vi "4461 - Create IO Channels Parallel Uneven.vi"(1 "Channels: Lockin":T1={"REF f (Hz)"=[0.4, 0.4], "REF phi (°)"=[0.0, 0.0]} {"REF phi (°)" format="%#_3g"}, 4 "sample mode":i32(ring)=10178 items=["Finite Samples"=10178, "Continuous Samples"=10123], 6 "sampling info":cluster{"Fs":dbl, "#s":dbl}, 7 "AI Buffer Size (S)":i32=10, 8 "error in":errorcluster, 9 "AO":T4={"AO amp (V)"=[0.1, 0.09, 0.08, 0.07, 0.06, 0.05, 0.04, 0.03], "AO DC (V)"=[0.0, 0.0, 0.0, 0.0, 0.0, 0.0, 0.0, 0.0], "AO f (Hz)"=[13.0, 13.0, 13.0, 13.0, 13.0, 13.0, 13.0, 13.0], "AO phi (°)"=[0.0, 0.0, 0.0, 0.0, 0.0, 0.0, 0.0, 0.0], "function"=[enum."Sine", enum."Sine", enum."Sine", enum."Sine", enum."Sine", enum."Sine", enum."Sine", enum."Sine"], "I+"=[]} {"AO f (Hz)" min=0.001 max=10000.0; "AO DC (V)" format="%.3p"; "AO amp (V)" format="%.3p"}, 10 "AO Configuration":T11, 11 "AI Configuration":T14) -> (0 "error out":errorcluster, 2 "AO Task":refnum<k21>[](array[refnum]), 3 "AI task":refnum<k21>[](array[refnum]), 5 "phase log":dbl[](array[numeric])=[0.99999999999938, 0.99999999999938])   [LabVIEW 2016]
uses:
  Instrument.Lockin/Typedefs/AI.config-array.ctl
  Instrument.Lockin/Typedefs/AI.config-cluster.ctl
  Instrument.Lockin/Typedefs/AI.coupling-enum.ctl
  Instrument.Lockin/Typedefs/446xAI-enum.ctl
  Instrument.Lockin/Typedefs/AO.config-array.ctl
  Instrument.Lockin/Typedefs/AO.config-cluster.ctl
  Instrument.Lockin/Typedefs/446xAO-enum.ctl
  Instrument.Lockin/Typedefs/AO-cluster.ctl
  Instrument.Lockin/Typedefs/AO_Amp-array.ctl
  Instrument.Lockin/Typedefs/AO_DC-array.ctl
  Instrument.Lockin/Typedefs/AO_f-array.ctl
  Instrument.Lockin/Typedefs/AO_phi-array.ctl
  Instrument.Lockin/Typedefs/Function-array.ctl
  Instrument.Lockin/Typedefs/Function-enum.ctl
  Instrument.Lockin/Typedefs/REF-cluster.ctl
  Instrument.Lockin/Typedefs/REF_f-array.ctl
  Instrument.Lockin/Typedefs/REF_phi-array.ctl
  <vilib>/DAQmx/write.llb/DAQmx Write (Analog 1D Wfm NChan NSamp).vi
  <vilib>/DAQmx/read.llb/DAQmx Read (Analog 1D Wfm NChan NSamp).vi
  <vilib>/DAQmx/create/channels.llb/DAQmx Create Channel (AI-Voltage-Basic).vi
  <vilib>/DAQmx/configure/timing.llb/DAQmx Timing (Sample Clock).vi
  <vilib>/DAQmx/create/channels.llb/DAQmx Create Channel (AO-Voltage-Basic).vi
  <vilib>/DAQmx/configure/trigger.llb/DAQmx Start Trigger (Digital Edge).vi
  <vilib>/DAQmx/miscellaneous.llb/DAQmx Fill In Error Info.vi
  <resource>/objmgr/daqmx.rc
  Instrument.Lockin/Instrument.Lockin.lvclass
panel:
  in  "AI.FilterDelay":dbl
  in  "AI.Gain":dbl
  in  "input terminal configuration":i32(ring)=-1 items=["default"=-1, "RSE"=10083, "NRSE"=10078, "Differential"=10106, "Pseudodifferential"=12529]
  in  "output terminal configuration":i32(ring)=-1 items=["Default"=-1, "RSE"=10083, "Differential"=10106, "Pseudodifferential"=12529]
  in  "SampClk.Timebase.Rate":dbl
  in  "SampQuant.SampPerChan":dbl
  # "1"
  # "2"
  # "3"
  # "4"
  # "5"
  # "6"
  # "7"
  # "8"
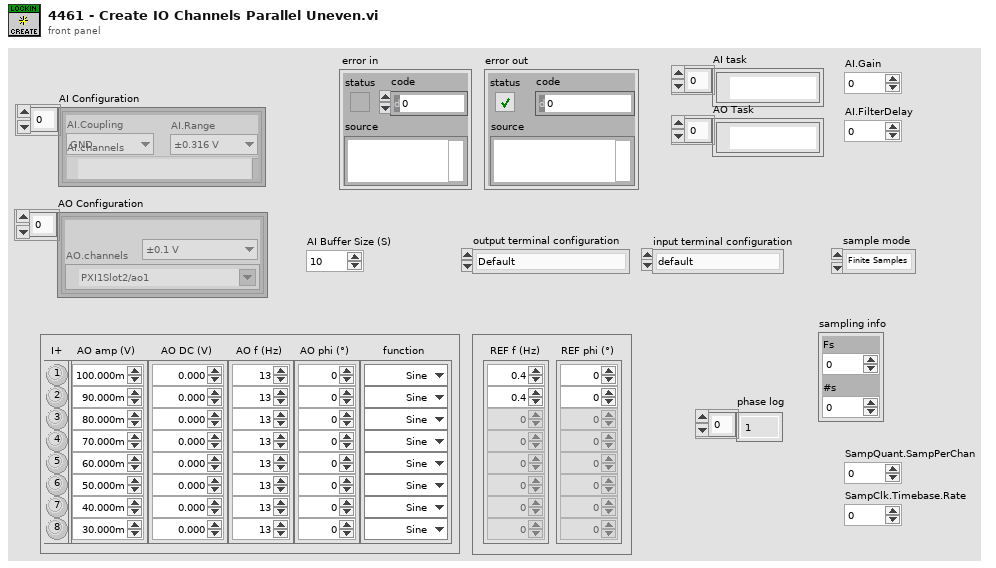
[diagram p1: front panel]
types:
  T1 = typedef "Instrument.Lockin.lvclass/REF-cluster.ctl" = cluster{"REF f (Hz)":T2, "REF phi (°)":T3}
  T2 = typedef "Instrument.Lockin.lvclass/REF_f-array.ctl" = dbl[]
  T3 = typedef "Instrument.Lockin.lvclass/REF_phi-array.ctl" = dbl[]
  T4 = typedef "Instrument.Lockin.lvclass/AO-cluster.ctl" = cluster{"AO amp (V)":T5, "AO DC (V)":T6, "AO f (Hz)":T7, "AO phi (°)":T8, "function":T9, "I+":bool[]}
  T5 = typedef "Instrument.Lockin.lvclass/AO_Amp-array.ctl" = dbl[]
  T6 = typedef "Instrument.Lockin.lvclass/AO_DC-array.ctl" = dbl[]
  T7 = typedef "Instrument.Lockin.lvclass/AO_f-array.ctl" = dbl[]
  T8 = typedef "Instrument.Lockin.lvclass/AO_phi-array.ctl" = dbl[]
  T9 = typedef "Instrument.Lockin.lvclass/Function-array.ctl" = T10[]
  T10 = typedef "Instrument.Lockin.lvclass/Function-enum.ctl" = enum16{"Sine", "Triangle", "Square", "Sawtooth"}
  T11 = typedef "Instrument.Lockin.lvclass/AO.config-array.ctl" = T12[]
  T12 = typedef "Instrument.Lockin.lvclass/AO.config-cluster.ctl" = cluster{"AO.Range":T13, "AO.channels":tag}
  T13 = typedef "Instrument.Lockin.lvclass/446xAO-enum.ctl" = enum16{"±0.1 V", "±1.0 V", "±10.0 V"}
  T14 = typedef "Instrument.Lockin.lvclass/AI.config-array.ctl" = T15[]
  T15 = typedef "Instrument.Lockin.lvclass/AI.config-cluster.ctl" = cluster{"AI.Coupling":T16, "AI.channels":tag, "AI.Range":T17}
  T16 = typedef "Instrument.Lockin.lvclass/AI.coupling-enum.ctl" = enum16{"AC", "DC", "GND"}
  T17 = typedef "Instrument.Lockin.lvclass/446xAI-enum.ctl" = enum16{"±0.316 V", "±1.00 V", "±3.16 V", "±10.0 V", "±31.6 V", "±42.4 V"}
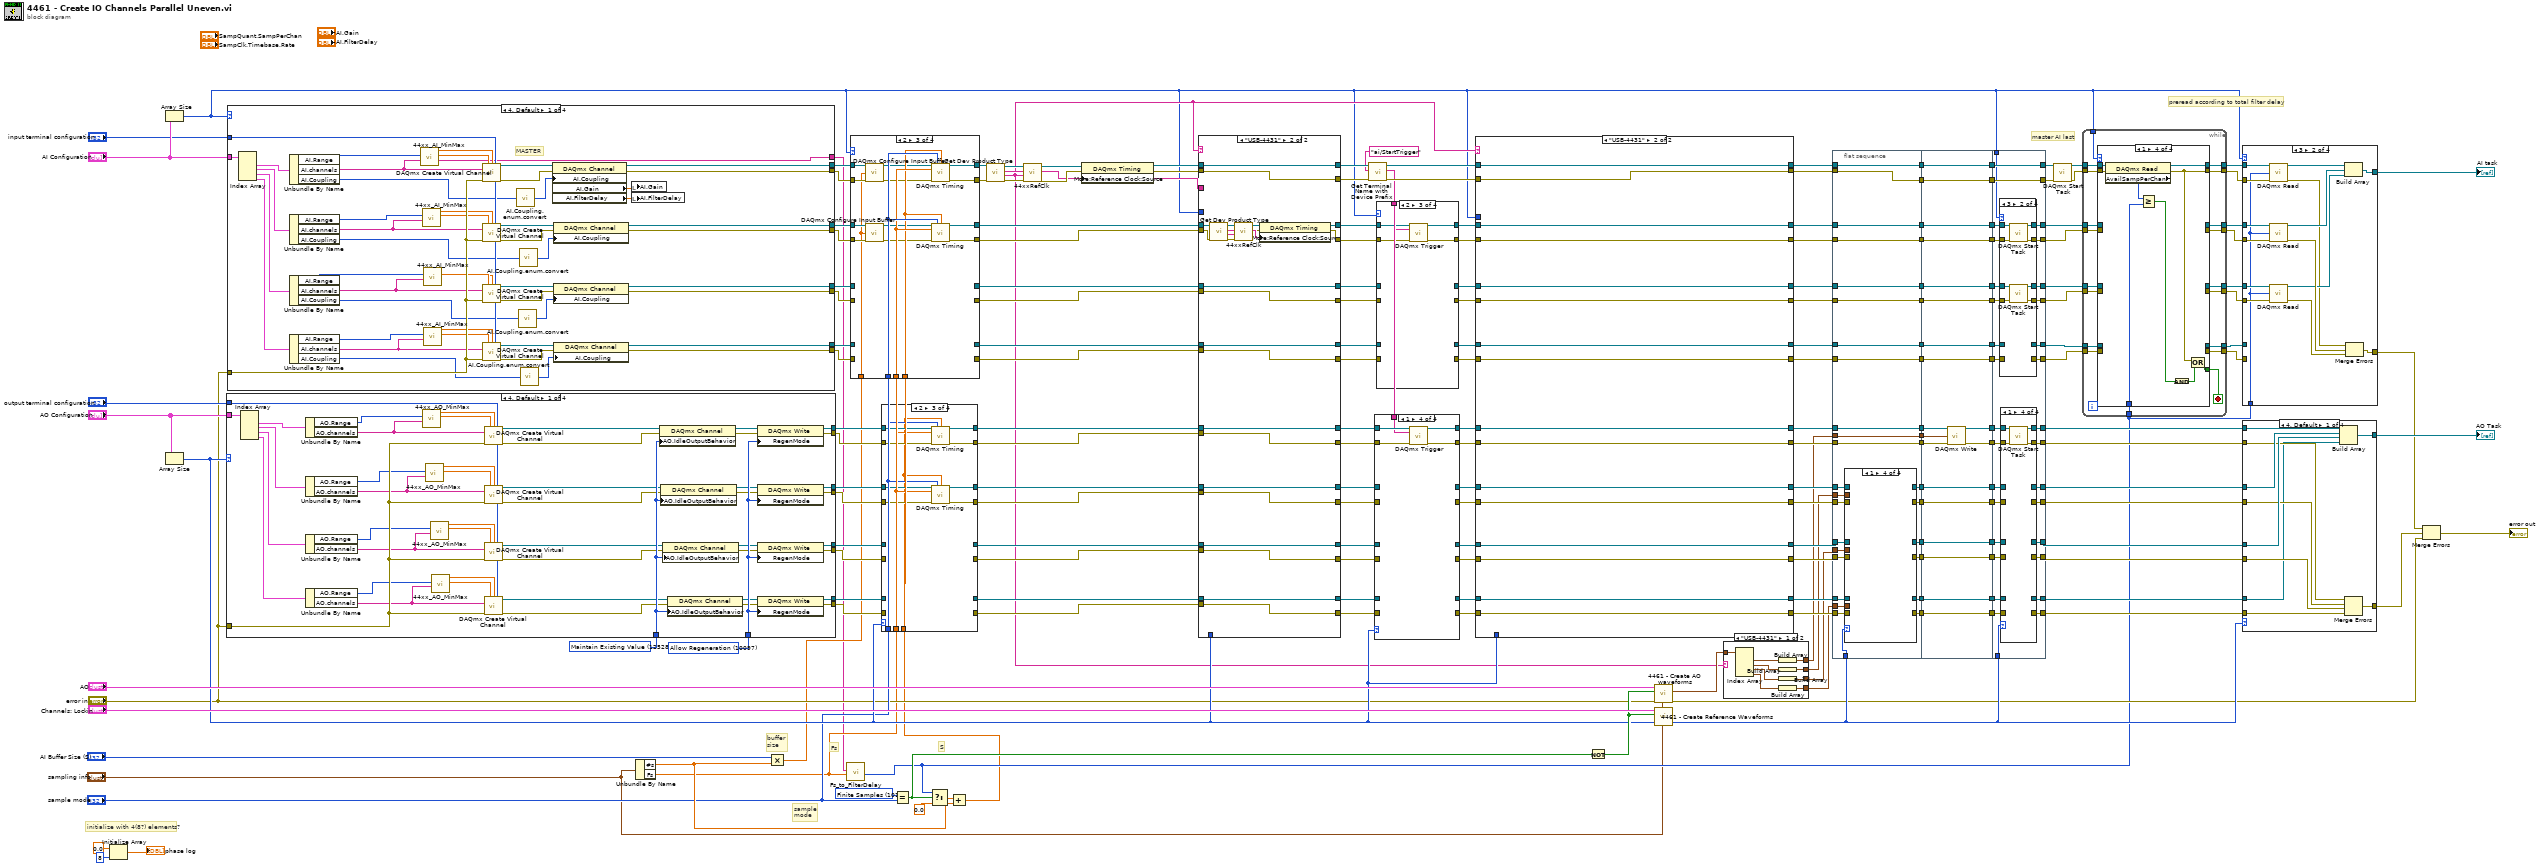
[diagram p0: block diagram]
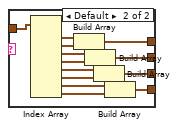
[diagram p2: hidden frame]
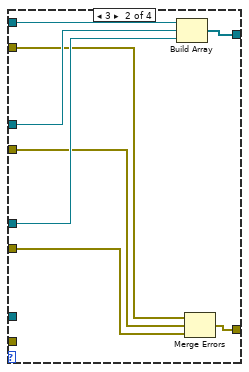
[diagram p3: hidden frame]
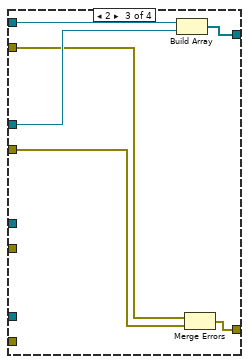
[diagram p4: hidden frame]
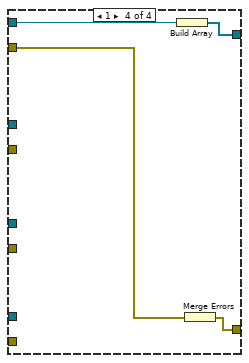
[diagram p5: hidden frame]
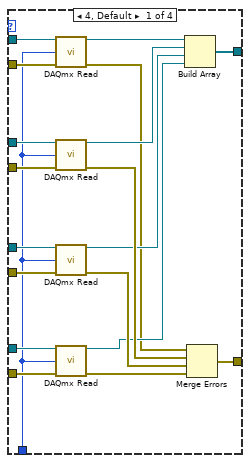
[diagram p6: hidden frame]
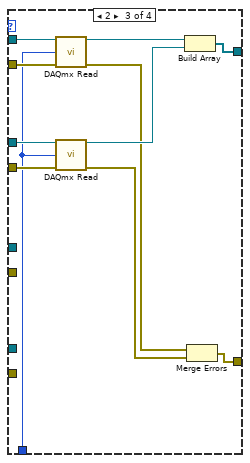
[diagram p7: hidden frame]
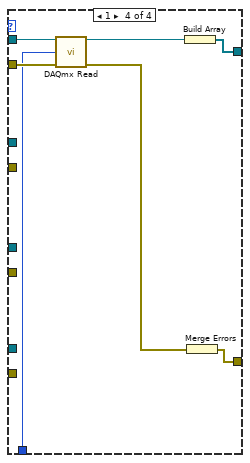
[diagram p8: hidden frame]
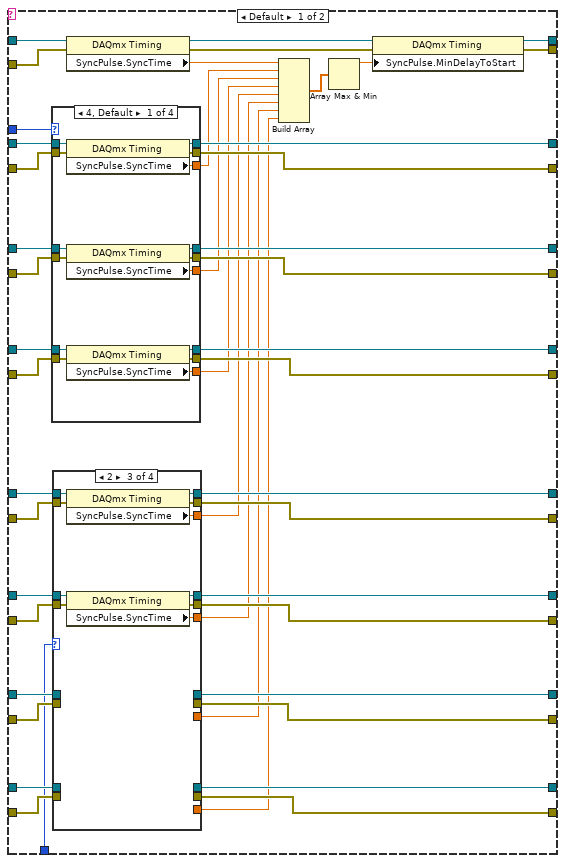
[diagram p9: hidden frame]
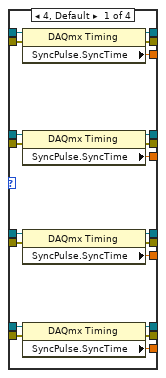
[diagram p10: hidden frame]
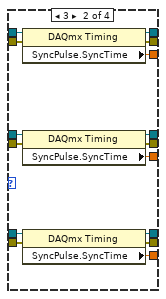
[diagram p11: hidden frame]
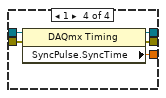
[diagram p12: hidden frame]
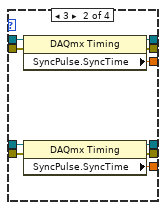
[diagram p13: hidden frame]
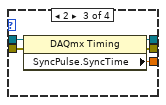
[diagram p14: hidden frame]
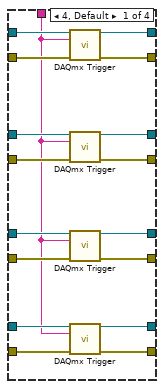
[diagram p16: hidden frame]
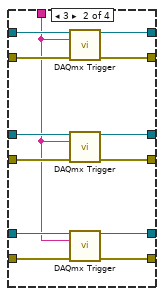
[diagram p17: hidden frame]
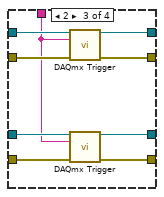
[diagram p18: hidden frame]
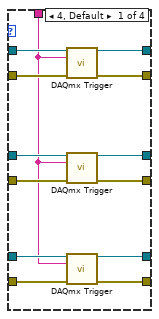
[diagram p19: hidden frame]
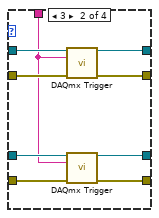
[diagram p20: hidden frame]
diagram:
  w173 = 10097 items=["Allow Regeneration"=10097, "Do Not Allow Regeneration"=10158] ("RegenMode")
  w175 = 12528 items=["Zero Volts"=12526, "High-Impedance"=12527, "Maintain Existing Value"=12528] ("AO.IdleOutputBehavior")
  w177 = 10178 items=["Finite Samples"=10178, "Continuous Samples"=10123] ("sample mode 2")
  # "preread according to total filter delay"
  # "master AI last"
  # "S"
  # "Fs"
  # "sample\nmode"
  # "buffer\nsize"
  # "initialize with 4(8?) elements?"
  n1 = Initialize Array(0.0 ("element"), 8 ("dimension size")) -> (→"phase log":dbl[])
  n2 = Array Size(array="AI Configuration") -> (size(s)=w6:i32)
  n3 = Array Size(array="AO Configuration") -> (size(s)=w168:i32)
  n4 = case shown="4, Default" w168 {
    tunnel: "AO Configuration" -> [w238 w276 w303 w319]
    tunnel: "error in" -> [w206 w251 w285 w308]
    tunnel: "output terminal configuration" -> [w233 w272 w300 w317]
    tunnel: [w228 w267 w295 w312] -> w84
    tunnel: [w227 _ _ _] -> w83
    tunnel: [w226 w266 w294 _] -> w82
    tunnel: [w225 w265 _ _] -> w81
    tunnel: w175 -> [w224 w264 w293 w311]
    tunnel: [w223 w263 w292 w310] -> w72
    tunnel: [w222 w262 w291 _] -> w71
    tunnel: [w221 w261 _ _] -> w70
    tunnel: [w220 _ _ _] -> w69
    tunnel: w173 -> [w219 w260 w290 w309]
    frame 4, Default {
      n5 = Index Array(array=w238) -> (element #1=w237:T12, element #2=w234:T12, element #3=w235:T12, element #4=w236:T12)  [unwired: 4 in]
      n6 = Unbundle By Name(w237) -> ("AO.Range"=w205:T13, "AO.channels"=w193:tag)
      n7 = Unbundle By Name(w234) -> ("AO.Range"=w200:T13, "AO.channels"=w192:tag)
      n8 = Unbundle By Name(w235) -> ("AO.Range"=w201:T13, "AO.channels"=w191:tag)
      n9 = Unbundle By Name(w236) -> ("AO.Range"=w202:T13, "AO.channels"=w190:tag)
      n10 = call "44xx_AO_MinMax.vi"("AO.channels"=w193, "AO.Range"=w205) -> ("AO.max"=w204:dbl, "AO.min"=w203:dbl)  [unwired: 7 in, 1 out]
      n11 = call "44xx_AO_MinMax.vi"("AO.channels"=w192, "AO.Range"=w200) -> ("AO.max"=w199:dbl, "AO.min"=w198:dbl)  [unwired: 7 in, 1 out]
      n12 = call "44xx_AO_MinMax.vi"("AO.channels"=w191, "AO.Range"=w201) -> ("AO.max"=w197:dbl, "AO.min"=w196:dbl)  [unwired: 7 in, 1 out]
      n13 = call "44xx_AO_MinMax.vi"("AO.channels"=w190, "AO.Range"=w202) -> ("AO.max"=w195:dbl, "AO.min"=w194:dbl)  [unwired: 7 in, 1 out]
      n14 = call-poly <vilib>:"DAQmx Create Virtual Channel.vi"("maximum value"=w204, "minimum value"=w203, "output terminal configuration"=w233, "physical channels"=w193, "error in"=w206) -> ("task out"=w232:refnum<k21>, "error out"=w231:errorcluster)  [unwired: 9 in]
      n15 = call-poly <vilib>:"DAQmx Create Virtual Channel.vi"("maximum value"=w199, "minimum value"=w198, "output terminal configuration"=w233, "physical channels"=w192, "error in"=w206) -> ("task out"=w213:refnum<k21>, "error out"=w214:errorcluster)  [unwired: 9 in]
      n16 = call-poly <vilib>:"DAQmx Create Virtual Channel.vi"("maximum value"=w197, "minimum value"=w196, "output terminal configuration"=w233, "physical channels"=w191, "error in"=w206) -> ("task out"=w215:refnum<k21>, "error out"=w216:errorcluster)  [unwired: 9 in]
      n17 = call-poly <vilib>:"DAQmx Create Virtual Channel.vi"("maximum value"=w195, "minimum value"=w194, "output terminal configuration"=w233, "physical channels"=w190, "error in"=w206) -> ("task out"=w218:refnum<k21>, "error out"=w217:errorcluster)  [unwired: 9 in]
      n18 = property class="DAQmx Channel"(reference=w232, error in=w231, "AO.IdleOutputBehavior"=w224) -> (reference out=w230:refnum<k21>, error out=w229:errorcluster)
      n19 = property class="DAQmx Channel"(reference=w213, error in=w214, "AO.IdleOutputBehavior"=w224) -> (reference out=w207:refnum<k21>, error out=w208:errorcluster)
      n20 = property class="DAQmx Channel"(reference=w215, error in=w216, "AO.IdleOutputBehavior"=w224) -> (reference out=w209:refnum<k21>, error out=w210:errorcluster)
      n21 = property class="DAQmx Channel"(reference=w218, error in=w217, "AO.IdleOutputBehavior"=w224) -> (reference out=w212:refnum<k21>, error out=w211:errorcluster)
      n22 = property class="DAQmx Write"(reference=w230, error in=w229, "RegenMode"=w219) -> (reference out=w228:refnum<k21>, error out=w223:errorcluster)
      n23 = property class="DAQmx Write"(reference=w207, error in=w208, "RegenMode"=w219) -> (reference out=w226:refnum<k21>, error out=w222:errorcluster)
      n24 = property class="DAQmx Write"(reference=w209, error in=w210, "RegenMode"=w219) -> (reference out=w225:refnum<k21>, error out=w221:errorcluster)
      n25 = property class="DAQmx Write"(reference=w212, error in=w211, "RegenMode"=w219) -> (reference out=w227:refnum<k21>, error out=w220:errorcluster)
    }
    frame 3 {
      n26 = Index Array(array=w276) -> (element #1=w275:T12, element #2=w273:T12, element #3=w274:T12)  [unwired: 4 in, 1 out]
      n27 = Unbundle By Name(w275) -> ("AO.Range"=w250:T13, "AO.channels"=w239:tag)
      n28 = Unbundle By Name(w273) -> ("AO.Range"=w246:T13, "AO.channels"=w240:tag)
      n29 = Unbundle By Name(w274) -> ("AO.Range"=w247:T13, "AO.channels"=w241:tag)
      n30 = call "44xx_AO_MinMax.vi"("AO.channels"=w239, "AO.Range"=w250) -> ("AO.max"=w249:dbl, "AO.min"=w248:dbl)  [unwired: 7 in, 1 out]
      n31 = call "44xx_AO_MinMax.vi"("AO.channels"=w240, "AO.Range"=w246) -> ("AO.max"=w245:dbl, "AO.min"=w244:dbl)  [unwired: 7 in, 1 out]
      n32 = call "44xx_AO_MinMax.vi"("AO.channels"=w241, "AO.Range"=w247) -> ("AO.max"=w243:dbl, "AO.min"=w242:dbl)  [unwired: 7 in, 1 out]
      n33 = call-poly <vilib>:"DAQmx Create Virtual Channel.vi"("maximum value"=w249, "minimum value"=w248, "output terminal configuration"=w272, "physical channels"=w239, "error in"=w251) -> ("task out"=w271:refnum<k21>, "error out"=w270:errorcluster)  [unwired: 9 in]
      n34 = call-poly <vilib>:"DAQmx Create Virtual Channel.vi"("maximum value"=w245, "minimum value"=w244, "output terminal configuration"=w272, "physical channels"=w240, "error in"=w251) -> ("task out"=w256:refnum<k21>, "error out"=w257:errorcluster)  [unwired: 9 in]
      n35 = call-poly <vilib>:"DAQmx Create Virtual Channel.vi"("maximum value"=w243, "minimum value"=w242, "output terminal configuration"=w272, "physical channels"=w241, "error in"=w251) -> ("task out"=w258:refnum<k21>, "error out"=w259:errorcluster)  [unwired: 9 in]
      n36 = property class="DAQmx Channel"(reference=w271, error in=w270, "AO.IdleOutputBehavior"=w264) -> (reference out=w269:refnum<k21>, error out=w268:errorcluster)
      n37 = property class="DAQmx Channel"(reference=w256, error in=w257, "AO.IdleOutputBehavior"=w264) -> (reference out=w252:refnum<k21>, error out=w253:errorcluster)
      n38 = property class="DAQmx Channel"(reference=w258, error in=w259, "AO.IdleOutputBehavior"=w264) -> (reference out=w254:refnum<k21>, error out=w255:errorcluster)
      n39 = property class="DAQmx Write"(reference=w269, error in=w268, "RegenMode"=w260) -> (reference out=w267:refnum<k21>, error out=w263:errorcluster)
      n40 = property class="DAQmx Write"(reference=w252, error in=w253, "RegenMode"=w260) -> (reference out=w266:refnum<k21>, error out=w262:errorcluster)
      n41 = property class="DAQmx Write"(reference=w254, error in=w255, "RegenMode"=w260) -> (reference out=w265:refnum<k21>, error out=w261:errorcluster)
    }
    frame 2 {
      n42 = Index Array(array=w303) -> (element #1=w302:T12, element #2=w301:T12)  [unwired: 4 in, 2 out]
      n43 = Unbundle By Name(w302) -> ("AO.Range"=w284:T13, "AO.channels"=w278:tag)
      n44 = Unbundle By Name(w301) -> ("AO.Range"=w281:T13, "AO.channels"=w277:tag)
      n45 = call "44xx_AO_MinMax.vi"("AO.channels"=w278, "AO.Range"=w284) -> ("AO.max"=w283:dbl, "AO.min"=w282:dbl)  [unwired: 7 in, 1 out]
      n46 = call "44xx_AO_MinMax.vi"("AO.channels"=w277, "AO.Range"=w281) -> ("AO.max"=w280:dbl, "AO.min"=w279:dbl)  [unwired: 7 in, 1 out]
      n47 = call-poly <vilib>:"DAQmx Create Virtual Channel.vi"("maximum value"=w283, "minimum value"=w282, "output terminal configuration"=w300, "physical channels"=w278, "error in"=w285) -> ("task out"=w299:refnum<k21>, "error out"=w298:errorcluster)  [unwired: 9 in]
      n48 = call-poly <vilib>:"DAQmx Create Virtual Channel.vi"("maximum value"=w280, "minimum value"=w279, "output terminal configuration"=w300, "physical channels"=w277, "error in"=w285) -> ("task out"=w288:refnum<k21>, "error out"=w289:errorcluster)  [unwired: 9 in]
      n49 = property class="DAQmx Channel"(reference=w299, error in=w298, "AO.IdleOutputBehavior"=w293) -> (reference out=w297:refnum<k21>, error out=w296:errorcluster)
      n50 = property class="DAQmx Channel"(reference=w288, error in=w289, "AO.IdleOutputBehavior"=w293) -> (reference out=w286:refnum<k21>, error out=w287:errorcluster)
      n51 = property class="DAQmx Write"(reference=w297, error in=w296, "RegenMode"=w290) -> (reference out=w295:refnum<k21>, error out=w292:errorcluster)
      n52 = property class="DAQmx Write"(reference=w286, error in=w287, "RegenMode"=w290) -> (reference out=w294:refnum<k21>, error out=w291:errorcluster)
    }
    frame 1 {
      n53 = Index Array(array=w319) -> (element #1=w318:T12)  [unwired: 4 in, 3 out]
      n54 = Unbundle By Name(w318) -> ("AO.Range"=w305:T13, "AO.channels"=w304:tag)
      n55 = call "44xx_AO_MinMax.vi"("AO.channels"=w304, "AO.Range"=w305) -> ("AO.max"=w307:dbl, "AO.min"=w306:dbl)  [unwired: 7 in, 1 out]
      n56 = call-poly <vilib>:"DAQmx Create Virtual Channel.vi"("maximum value"=w307, "minimum value"=w306, "output terminal configuration"=w317, "physical channels"=w304, "error in"=w308) -> ("task out"=w316:refnum<k21>, "error out"=w315:errorcluster)  [unwired: 9 in]
      n57 = property class="DAQmx Channel"(reference=w316, error in=w315, "AO.IdleOutputBehavior"=w311) -> (reference out=w314:refnum<k21>, error out=w313:errorcluster)
      n58 = property class="DAQmx Write"(reference=w314, error in=w313, "RegenMode"=w309) -> (reference out=w312:refnum<k21>, error out=w310:errorcluster)
    }
  }
  n59 = case shown="4, Default" w6 {
    tunnel: "AI Configuration" -> [w369 w408 w436 w453]
    tunnel: "error in" -> [w368 w407 w435 w452]
    tunnel: "input terminal configuration" -> [w367 w406 w434 w451]
    tunnel: [w366 w405 w433 _] -> w75
    tunnel: [w365 w404 _ _] -> w74
    tunnel: [w364 _ _ _] -> w73
    tunnel: [w363 w403 w432 _] -> w18
    tunnel: [w362 w402 _ _] -> w17
    tunnel: [w361 _ _ _] -> w16
    tunnel: [w360 w401 w431 w450] -> w48
    tunnel: [w359 w400 w430 w449] -> w19
    tunnel: [w320 w370 w409 w437] -> w2
    frame 4, Default {
      # "MASTER"
      n60 = Index Array(array=w369) -> (element #1=w334:T15, element #2=w356:T15, element #3=w355:T15, element #4=w354:T15)  [unwired: 4 in]
      n61 = Unbundle By Name(w334) -> ("AI.Range"=w335:T17, "AI.channels"=w326:tag, "AI.Coupling"=w351:T16)
      n62 = Unbundle By Name(w356) -> ("AI.Range"=w324:T17, "AI.channels"=w325:tag, "AI.Coupling"=w342:T16)
      n63 = Unbundle By Name(w355) -> ("AI.Range"=w333:T17, "AI.channels"=w323:tag, "AI.Coupling"=w343:T16)
      n64 = Unbundle By Name(w354) -> ("AI.Range"=w322:T17, "AI.channels"=w321:tag, "AI.Coupling"=w344:T16)
      n65 = call "44xx_AI_MinMax.vi"("AI.channels"=w326, "446x AI"=w335) -> ("ProductType"=w320:string, "AI.Max"=w337:dbl, "AI.Min"=w336:dbl)  [unwired: 7 in]
      n66 = call "44xx_AI_MinMax.vi"("AI.channels"=w325, "446x AI"=w324) -> ("AI.Max"=w332:dbl, "AI.Min"=w329:dbl)  [unwired: 7 in, 1 out]
      n67 = call "44xx_AI_MinMax.vi"("AI.channels"=w321, "446x AI"=w322) -> ("AI.Max"=w328:dbl, "AI.Min"=w327:dbl)  [unwired: 7 in, 1 out]
      n68 = call "44xx_AI_MinMax.vi"("AI.channels"=w323, "446x AI"=w333) -> ("AI.Max"=w331:dbl, "AI.Min"=w330:dbl)  [unwired: 7 in, 1 out]
      n69 = call-poly <vilib>:"DAQmx Create Virtual Channel.vi"("maximum value"=w337, "minimum value"=w336, "input terminal configuration"=w367, "physical channels"=w326, "error in"=w368) -> ("task out"=w358:refnum<k21>, "error out"=w357:errorcluster)  [unwired: 9 in]
      n70 = call-poly <vilib>:"DAQmx Create Virtual Channel.vi"("maximum value"=w332, "minimum value"=w329, "input terminal configuration"=w367, "physical channels"=w325, "error in"=w368) -> ("task out"=w349:refnum<k21>, "error out"=w350:errorcluster)  [unwired: 9 in]
      n71 = call-poly <vilib>:"DAQmx Create Virtual Channel.vi"("maximum value"=w331, "minimum value"=w330, "input terminal configuration"=w367, "physical channels"=w323, "error in"=w368) -> ("task out"=w348:refnum<k21>, "error out"=w347:errorcluster)  [unwired: 9 in]
      n72 = call-poly <vilib>:"DAQmx Create Virtual Channel.vi"("maximum value"=w328, "minimum value"=w327, "input terminal configuration"=w367, "physical channels"=w321, "error in"=w368) -> ("task out"=w345:refnum<k21>, "error out"=w346:errorcluster)  [unwired: 9 in]
      n73 = call "AI.Coupling.enum.convert.vi"("AI.Coupling"=w351) -> ("Numeric"=w341:i32)
      n74 = call "AI.Coupling.enum.convert.vi"("AI.Coupling"=w343) -> ("Numeric"=w339:i32)
      n75 = call "AI.Coupling.enum.convert.vi"("AI.Coupling"=w342) -> ("Numeric"=w340:i32)
      n76 = call "AI.Coupling.enum.convert.vi"("AI.Coupling"=w344) -> ("Numeric"=w338:i32)
      n77 = property class="DAQmx Channel"(reference=w358, error in=w357, "AI.Coupling"=w341) -> (reference out=w360:refnum<k21>, error out=w359:errorcluster, "AI.Gain"=w353:dbl, "AI.FilterDelay"=w352:dbl)
      n78 = property class="DAQmx Channel"(reference=w349, error in=w350, "AI.Coupling"=w340) -> (reference out=w366:refnum<k21>, error out=w363:errorcluster)
      n79 = property class="DAQmx Channel"(reference=w348, error in=w347, "AI.Coupling"=w339) -> (reference out=w365:refnum<k21>, error out=w362:errorcluster)
      n80 = property class="DAQmx Channel"(reference=w345, error in=w346, "AI.Coupling"=w338) -> (reference out=w364:refnum<k21>, error out=w361:errorcluster)
      n81 = local write "AI.Gain"(w353) -> ()
      n82 = local write "AI.FilterDelay"(w352) -> ()
    }
    frame 3 {
      # "MASTER"
      n83 = Index Array(array=w408) -> (element #1=w380:T15, element #2=w397:T15, element #3=w396:T15)  [unwired: 4 in, 1 out]
      n84 = Unbundle By Name(w380) -> ("AI.Range"=w381:T17, "AI.channels"=w371:tag, "AI.Coupling"=w393:T16)
      n85 = Unbundle By Name(w397) -> ("AI.Range"=w372:T17, "AI.channels"=w373:tag, "AI.Coupling"=w387:T16)
      n86 = Unbundle By Name(w396) -> ("AI.Range"=w379:T17, "AI.channels"=w374:tag, "AI.Coupling"=w388:T16)
      n87 = call "44xx_AI_MinMax.vi"("AI.channels"=w371, "446x AI"=w381) -> ("ProductType"=w370:string, "AI.Max"=w383:dbl, "AI.Min"=w382:dbl)  [unwired: 7 in]
      n88 = call "44xx_AI_MinMax.vi"("AI.channels"=w373, "446x AI"=w372) -> ("AI.Max"=w378:dbl, "AI.Min"=w375:dbl)  [unwired: 7 in, 1 out]
      n89 = call "44xx_AI_MinMax.vi"("AI.channels"=w374, "446x AI"=w379) -> ("AI.Max"=w377:dbl, "AI.Min"=w376:dbl)  [unwired: 7 in, 1 out]
      n90 = call-poly <vilib>:"DAQmx Create Virtual Channel.vi"("maximum value"=w383, "minimum value"=w382, "input terminal configuration"=w406, "physical channels"=w371, "error in"=w407) -> ("task out"=w399:refnum<k21>, "error out"=w398:errorcluster)  [unwired: 9 in]
      n91 = call-poly <vilib>:"DAQmx Create Virtual Channel.vi"("maximum value"=w378, "minimum value"=w375, "input terminal configuration"=w406, "physical channels"=w373, "error in"=w407) -> ("task out"=w391:refnum<k21>, "error out"=w392:errorcluster)  [unwired: 9 in]
      n92 = call-poly <vilib>:"DAQmx Create Virtual Channel.vi"("maximum value"=w377, "minimum value"=w376, "input terminal configuration"=w406, "physical channels"=w374, "error in"=w407) -> ("task out"=w390:refnum<k21>, "error out"=w389:errorcluster)  [unwired: 9 in]
      n93 = call "AI.Coupling.enum.convert.vi"("AI.Coupling"=w393) -> ("Numeric"=w386:i32)
      n94 = call "AI.Coupling.enum.convert.vi"("AI.Coupling"=w388) -> ("Numeric"=w384:i32)
      n95 = call "AI.Coupling.enum.convert.vi"("AI.Coupling"=w387) -> ("Numeric"=w385:i32)
      n96 = property class="DAQmx Channel"(reference=w399, error in=w398, "AI.Coupling"=w386) -> (reference out=w401:refnum<k21>, error out=w400:errorcluster, "AI.Gain"=w395:dbl, "AI.FilterDelay"=w394:dbl)
      n97 = property class="DAQmx Channel"(reference=w391, error in=w392, "AI.Coupling"=w385) -> (reference out=w405:refnum<k21>, error out=w403:errorcluster)
      n98 = property class="DAQmx Channel"(reference=w390, error in=w389, "AI.Coupling"=w384) -> (reference out=w404:refnum<k21>, error out=w402:errorcluster)
      n99 = local write "AI.Gain"(w395) -> ()
      n100 = local write "AI.FilterDelay"(w394) -> ()
    }
    frame 2 {
      # "MASTER"
      n101 = Index Array(array=w436) -> (element #1=w415:T15, element #2=w427:T15)  [unwired: 4 in, 2 out]
      n102 = Unbundle By Name(w415) -> ("AI.Range"=w416:T17, "AI.channels"=w410:tag, "AI.Coupling"=w424:T16)
      n103 = Unbundle By Name(w427) -> ("AI.Range"=w412:T17, "AI.channels"=w411:tag, "AI.Coupling"=w421:T16)
      n104 = call "44xx_AI_MinMax.vi"("AI.channels"=w410, "446x AI"=w416) -> ("ProductType"=w409:string, "AI.Max"=w418:dbl, "AI.Min"=w417:dbl)  [unwired: 7 in]
      n105 = call "44xx_AI_MinMax.vi"("AI.channels"=w411, "446x AI"=w412) -> ("AI.Max"=w414:dbl, "AI.Min"=w413:dbl)  [unwired: 7 in, 1 out]
      n106 = call-poly <vilib>:"DAQmx Create Virtual Channel.vi"("maximum value"=w418, "minimum value"=w417, "input terminal configuration"=w434, "physical channels"=w410, "error in"=w435) -> ("task out"=w429:refnum<k21>, "error out"=w428:errorcluster)  [unwired: 9 in]
      n107 = call-poly <vilib>:"DAQmx Create Virtual Channel.vi"("maximum value"=w414, "minimum value"=w413, "input terminal configuration"=w434, "physical channels"=w411, "error in"=w435) -> ("task out"=w422:refnum<k21>, "error out"=w423:errorcluster)  [unwired: 9 in]
      n108 = call "AI.Coupling.enum.convert.vi"("AI.Coupling"=w424) -> ("Numeric"=w420:i32)
      n109 = call "AI.Coupling.enum.convert.vi"("AI.Coupling"=w421) -> ("Numeric"=w419:i32)
      n110 = property class="DAQmx Channel"(reference=w429, error in=w428, "AI.Coupling"=w420) -> (reference out=w431:refnum<k21>, error out=w430:errorcluster, "AI.Gain"=w426:dbl, "AI.FilterDelay"=w425:dbl)
      n111 = property class="DAQmx Channel"(reference=w422, error in=w423, "AI.Coupling"=w419) -> (reference out=w433:refnum<k21>, error out=w432:errorcluster)
      n112 = local write "AI.Gain"(w426) -> ()
      n113 = local write "AI.FilterDelay"(w425) -> ()
    }
    frame 1 {
      # "MASTER"
      n114 = Index Array(array=w453) -> (element #1=w442:T15)  [unwired: 4 in, 3 out]
      n115 = Unbundle By Name(w442) -> ("AI.Range"=w441:T17, "AI.channels"=w440:tag, "AI.Coupling"=w444:T16)
      n116 = call "44xx_AI_MinMax.vi"("AI.channels"=w440, "446x AI"=w441) -> ("ProductType"=w437:string, "AI.Max"=w439:dbl, "AI.Min"=w438:dbl)  [unwired: 7 in]
      n117 = call-poly <vilib>:"DAQmx Create Virtual Channel.vi"("maximum value"=w439, "minimum value"=w438, "input terminal configuration"=w451, "physical channels"=w440, "error in"=w452) -> ("task out"=w448:refnum<k21>, "error out"=w447:errorcluster)  [unwired: 9 in]
      n118 = call "AI.Coupling.enum.convert.vi"("AI.Coupling"=w444) -> ("Numeric"=w443:i32)
      n119 = property class="DAQmx Channel"(reference=w448, error in=w447, "AI.Coupling"=w443) -> (reference out=w450:refnum<k21>, error out=w449:errorcluster, "AI.Gain"=w446:dbl, "AI.FilterDelay"=w445:dbl)
      n120 = local write "AI.Gain"(w446) -> ()
      n121 = local write "AI.FilterDelay"(w445) -> ()
    }
  }
  n122 = Unbundle By Name("sampling info") -> ("#s"=w174:dbl, "Fs"=w5:dbl)
  n123 = Multiply(x="AI Buffer Size (S)", y=w174) -> (x*y=w20:dbl)
  n124 = call "Fs_to_FilterDelay.vi"("Fs"=w5, "ProductType"=w2) -> ("Total Filter Delay (samples)"=w4:u32)  [unwired: 9 in]
  n125 = Equal?(x=w177, y="sample mode") -> (x = y?=w171:bool)
  n126 = Select(t=w4, s=w171, f=0.0) -> (s? t:f=w178:dbl)
  n127 = Add(x=w178, y=w174) -> (x+y=w3:dbl)
  n128 = case shown="2" w6 {
    tunnel: [w481 w503 w519 w529] -> w14
    tunnel: [w480 w502 w518 w528] -> w15
    tunnel: [w479 w501 w517 _] -> w131
    tunnel: [w478 w500 w516 _] -> w130
    tunnel: [w477 w499 _ _] -> w125
    tunnel: [w476 w498 _ _] -> w124
    tunnel: [w475 _ _ _] -> w123
    tunnel: [w474 _ _ _] -> w122
    tunnel: w73 -> [w464 _ _ _]
    tunnel: w74 -> [w466 w490 _ _]
    tunnel: w17 -> [w459 w487 _ _]
    tunnel: w16 -> [w465 _ _ _]
    tunnel: w18 -> [w468 w492 w510 _]
    tunnel: w75 -> [w467 w491 w509 _]
    tunnel: "sample mode" -> [w473 w497 w515 w527]
    tunnel: w5 -> [w472 w496 w514 w526]
    tunnel: w3 -> [w471 w495 w513 w525]
    tunnel: w19 -> [w470 w494 w512 w524]
    tunnel: w48 -> [w469 w493 w511 w523]
    tunnel: w20 -> [w454 w482 w504 w520]
    frame 4, Default {
      n129 = call <vilib>:"DAQmx Configure Input Buffer.vi"("task/channels in"=w469, "buffer size (in samples per channel)"=w454, "error in"=w470) -> ("task out"=w455:refnum<k21>, "error out"=w456:errorcluster)  [unwired: 11 in]
      n130 = call <vilib>:"DAQmx Configure Input Buffer.vi"("task/channels in"=w467, "buffer size (in samples per channel)"=w454, "error in"=w468) -> ("task out"=w457:refnum<k21>, "error out"=w458:errorcluster)  [unwired: 11 in]
      n131 = call <vilib>:"DAQmx Configure Input Buffer.vi"("task/channels in"=w466, "buffer size (in samples per channel)"=w454, "error in"=w459) -> ("task out"=w460:refnum<k21>, "error out"=w461:errorcluster)  [unwired: 11 in]
      n132 = call <vilib>:"DAQmx Configure Input Buffer.vi"("task/channels in"=w464, "buffer size (in samples per channel)"=w454, "error in"=w465) -> ("task out"=w463:refnum<k21>, "error out"=w462:errorcluster)  [unwired: 11 in]
      n133 = call-poly <vilib>:"DAQmx Timing.vi"("task/channels in"=w455, "sample mode"=w473, "samples per channel"=w471, "rate"=w472, "error in"=w456) -> ("task out"=w481:refnum<k21>, "error out"=w480:errorcluster)  [unwired: 9 in]
      n134 = call-poly <vilib>:"DAQmx Timing.vi"("task/channels in"=w457, "sample mode"=w473, "samples per channel"=w471, "rate"=w472, "error in"=w458) -> ("task out"=w479:refnum<k21>, "error out"=w478:errorcluster)  [unwired: 9 in]
      n135 = call-poly <vilib>:"DAQmx Timing.vi"("task/channels in"=w460, "sample mode"=w473, "samples per channel"=w471, "rate"=w472, "error in"=w461) -> ("task out"=w476:refnum<k21>, "error out"=w477:errorcluster)  [unwired: 9 in]
      n136 = call-poly <vilib>:"DAQmx Timing.vi"("task/channels in"=w463, "sample mode"=w473, "samples per channel"=w471, "rate"=w472, "error in"=w462) -> ("task out"=w475:refnum<k21>, "error out"=w474:errorcluster)  [unwired: 9 in]
    }
    frame 3 {
      n137 = call <vilib>:"DAQmx Configure Input Buffer.vi"("task/channels in"=w493, "buffer size (in samples per channel)"=w482, "error in"=w494) -> ("task out"=w483:refnum<k21>, "error out"=w484:errorcluster)  [unwired: 11 in]
      n138 = call <vilib>:"DAQmx Configure Input Buffer.vi"("task/channels in"=w491, "buffer size (in samples per channel)"=w482, "error in"=w492) -> ("task out"=w485:refnum<k21>, "error out"=w486:errorcluster)  [unwired: 11 in]
      n139 = call <vilib>:"DAQmx Configure Input Buffer.vi"("task/channels in"=w490, "buffer size (in samples per channel)"=w482, "error in"=w487) -> ("task out"=w488:refnum<k21>, "error out"=w489:errorcluster)  [unwired: 11 in]
      n140 = call-poly <vilib>:"DAQmx Timing.vi"("task/channels in"=w483, "sample mode"=w497, "samples per channel"=w495, "rate"=w496, "error in"=w484) -> ("task out"=w503:refnum<k21>, "error out"=w502:errorcluster)  [unwired: 9 in]
      n141 = call-poly <vilib>:"DAQmx Timing.vi"("task/channels in"=w485, "sample mode"=w497, "samples per channel"=w495, "rate"=w496, "error in"=w486) -> ("task out"=w501:refnum<k21>, "error out"=w500:errorcluster)  [unwired: 9 in]
      n142 = call-poly <vilib>:"DAQmx Timing.vi"("task/channels in"=w488, "sample mode"=w497, "samples per channel"=w495, "rate"=w496, "error in"=w489) -> ("task out"=w498:refnum<k21>, "error out"=w499:errorcluster)  [unwired: 9 in]
    }
    frame 2 {
      n143 = call <vilib>:"DAQmx Configure Input Buffer.vi"("task/channels in"=w511, "buffer size (in samples per channel)"=w504, "error in"=w512) -> ("task out"=w505:refnum<k21>, "error out"=w506:errorcluster)  [unwired: 11 in]
      n144 = call <vilib>:"DAQmx Configure Input Buffer.vi"("task/channels in"=w509, "buffer size (in samples per channel)"=w504, "error in"=w510) -> ("task out"=w507:refnum<k21>, "error out"=w508:errorcluster)  [unwired: 11 in]
      n145 = call-poly <vilib>:"DAQmx Timing.vi"("task/channels in"=w505, "sample mode"=w515, "samples per channel"=w513, "rate"=w514, "error in"=w506) -> ("task out"=w519:refnum<k21>, "error out"=w518:errorcluster)  [unwired: 9 in]
      n146 = call-poly <vilib>:"DAQmx Timing.vi"("task/channels in"=w507, "sample mode"=w515, "samples per channel"=w513, "rate"=w514, "error in"=w508) -> ("task out"=w517:refnum<k21>, "error out"=w516:errorcluster)  [unwired: 9 in]
    }
    frame 1 {
      n147 = call <vilib>:"DAQmx Configure Input Buffer.vi"("task/channels in"=w523, "buffer size (in samples per channel)"=w520, "error in"=w524) -> ("task out"=w521:refnum<k21>, "error out"=w522:errorcluster)  [unwired: 11 in]
      n148 = call-poly <vilib>:"DAQmx Timing.vi"("task/channels in"=w521, "sample mode"=w527, "samples per channel"=w525, "rate"=w526, "error in"=w522) -> ("task out"=w529:refnum<k21>, "error out"=w528:errorcluster)  [unwired: 9 in]
    }
  }
  n149 = case shown="2" w168 {
    tunnel: w84 -> [w548 w563 w574 w581]
    tunnel: w83 -> [w547 _ _ _]
    tunnel: w82 -> [w546 w562 w573 _]
    tunnel: w81 -> [w545 w561 _ _]
    tunnel: [w544 w560 w572 _] -> w80
    tunnel: [w543 _ _ _] -> w79
    tunnel: [w542 _ _ _] -> w78
    tunnel: [w541 w559 _ _] -> w77
    tunnel: [w540 w558 w571 w580] -> w76
    tunnel: "sample mode" -> [w539 w557 w570 w579]
    tunnel: w5 -> [w538 w556 w569 w578]
    tunnel: w3 -> [w530 w549 w564 w575]
    tunnel: w72 -> [w537 w555 w568 w577]
    tunnel: w71 -> [w536 w554 w567 _]
    tunnel: w70 -> [w535 w553 _ _]
    tunnel: w69 -> [w534 _ _ _]
    tunnel: [w533 w552 w566 w576] -> w32
    tunnel: [w532 w551 w565 _] -> w52
    tunnel: [w531 w550 _ _] -> w51
    frame 4, Default {
      n150 = call-poly <vilib>:"DAQmx Timing.vi"("task/channels in"=w548, "sample mode"=w539, "samples per channel"=w530, "rate"=w538, "error in"=w537) -> ("task out"=w540:refnum<k21>, "error out"=w533:errorcluster)  [unwired: 9 in]
      n151 = call-poly <vilib>:"DAQmx Timing.vi"("task/channels in"=w546, "sample mode"=w539, "samples per channel"=w530, "rate"=w538, "error in"=w536) -> ("task out"=w544:refnum<k21>, "error out"=w532:errorcluster)  [unwired: 9 in]
      n152 = call-poly <vilib>:"DAQmx Timing.vi"("task/channels in"=w545, "sample mode"=w539, "samples per channel"=w530, "rate"=w538, "error in"=w535) -> ("task out"=w541:refnum<k21>, "error out"=w531:errorcluster)  [unwired: 9 in]
      n153 = call-poly <vilib>:"DAQmx Timing.vi"("task/channels in"=w547, "sample mode"=w539, "samples per channel"=w530, "rate"=w538, "error in"=w534) -> ("task out"=w542:refnum<k21>, "error out"=w543:errorcluster)  [unwired: 9 in]
    }
    frame 3 {
      n154 = call-poly <vilib>:"DAQmx Timing.vi"("task/channels in"=w563, "sample mode"=w557, "samples per channel"=w549, "rate"=w556, "error in"=w555) -> ("task out"=w558:refnum<k21>, "error out"=w552:errorcluster)  [unwired: 9 in]
      n155 = call-poly <vilib>:"DAQmx Timing.vi"("task/channels in"=w562, "sample mode"=w557, "samples per channel"=w549, "rate"=w556, "error in"=w554) -> ("task out"=w560:refnum<k21>, "error out"=w551:errorcluster)  [unwired: 9 in]
      n156 = call-poly <vilib>:"DAQmx Timing.vi"("task/channels in"=w561, "sample mode"=w557, "samples per channel"=w549, "rate"=w556, "error in"=w553) -> ("task out"=w559:refnum<k21>, "error out"=w550:errorcluster)  [unwired: 9 in]
    }
    frame 2 {
      n157 = call-poly <vilib>:"DAQmx Timing.vi"("task/channels in"=w574, "sample mode"=w570, "samples per channel"=w564, "rate"=w569, "error in"=w568) -> ("task out"=w571:refnum<k21>, "error out"=w566:errorcluster)  [unwired: 9 in]
      n158 = call-poly <vilib>:"DAQmx Timing.vi"("task/channels in"=w573, "sample mode"=w570, "samples per channel"=w564, "rate"=w569, "error in"=w567) -> ("task out"=w572:refnum<k21>, "error out"=w565:errorcluster)  [unwired: 9 in]
    }
    frame 1 {
      n159 = call-poly <vilib>:"DAQmx Timing.vi"("task/channels in"=w581, "sample mode"=w579, "samples per channel"=w575, "rate"=w578, "error in"=w577) -> ("task out"=w580:refnum<k21>, "error out"=w576:errorcluster)  [unwired: 9 in]
    }
  }
  n160 = call "Get Dev Product Type.vi"("error in (no error)"=w15, "Refnum in"=w14) -> ("error out"=w9:errorcluster, "ProductType"=w8:string, "ActiveDev"=w13:tag, "Refnum out"=w12:refnum<k21>)  [unwired: 6 in]
  n161 = call "44xxRefClk.vi"("error in (no error)"=w9, "ProductType"=w8, "ActiveDev"=w13, "Refnum in"=w12) -> ("error out"=w10:errorcluster, "RefClk.Src"=w7:tag, "Refnum out"=w11:refnum<k21>)  [unwired: 5 in]
  n162 = property class="DAQmx Timing"(reference=w11, error in=w10, "More:Reference Clock:Source"=w7) -> (reference out=w91:refnum<k21>, error out=w33:errorcluster)
  n163 = case shown="\"USB-4431\"" w8 {
    tunnel: [w618 w721] -> w135
    tunnel: [w617 w720] -> w134
    tunnel: w131 -> [w616 w707]
    tunnel: w130 -> [w615 w703]
    tunnel: [w614 w697] -> w129
    tunnel: [w613 w698] -> w128
    tunnel: [w612 w718] -> w127
    tunnel: [w611 w719] -> w126
    tunnel: w125 -> [w610 w718]
    tunnel: w124 -> [w609 w719]
    tunnel: w123 -> [w608 w717]
    tunnel: w122 -> [w607 w716]
    tunnel: [w606 w717] -> w121
    tunnel: [w605 w716] -> w120
    tunnel: [w604 w715] -> w118
    tunnel: [w603 w714] -> w117
    tunnel: [w602 w712] -> w114
    tunnel: [w601 w713] -> w113
    tunnel: [w600 w711] -> w112
    tunnel: [w599 w710] -> w111
    tunnel: [w598 w708] -> w110
    tunnel: [w597 w709] -> w109
    tunnel: w91 -> [w596 w721]
    tunnel: w80 -> [w595 w713]
    tunnel: w79 -> [w594 w708]
    tunnel: w78 -> [w593 w709]
    tunnel: w77 -> [w592 w711]
    tunnel: w76 -> [w591 w715]
    tunnel: w52 -> [w589 w712]
    tunnel: w51 -> [w588 w710]
    tunnel: w33 -> [w585 w720]
    tunnel: w7 -> [w584 _]
    tunnel: w6 -> [w582 _]
    tunnel: w32 -> [w590 w714]
    tunnel: w168 -> [w583 _]
    frame Default {
      n164 = call "Get Terminal Name with Device Prefix.vi"("error in (no error)"=w585, "Local Terminal Name"="SyncPulse", "task/channels in"=w596) -> ("error out"=w617:errorcluster, "Terminal Name with Device Prefix"=w586:tag, "task out"=w618:refnum<k21>)  [unwired: 6 in]
      n165 = case shown="2" w583 {
        tunnel: [w636 w650 w660 w666] -> w604
        tunnel: [w635 w649 w659 w665] -> w603
        tunnel: [w634 w648 w658 _] -> w602
        tunnel: [w633 w647 w657 _] -> w601
        tunnel: [w632 w646 _ _] -> w600
        tunnel: [w631 w645 _ _] -> w599
        tunnel: [w630 _ _ _] -> w598
        tunnel: [w629 _ _ _] -> w597
        tunnel: w595 -> [w628 w644 w656 _]
        tunnel: w594 -> [w627 _ _ _]
        tunnel: w593 -> [w626 _ _ _]
        tunnel: w592 -> [w625 w643 _ _]
        tunnel: w591 -> [w624 w642 w655 w664]
        tunnel: w590 -> [w623 w641 w654 w663]
        tunnel: w589 -> [w622 w640 w653 _]
        tunnel: w588 -> [w621 w639 _ _]
        tunnel: w586 -> [w620 w638 w652 w662]
        tunnel: w584 -> [w619 w637 w651 w661]
        frame 4, Default {
          n166 = property class="DAQmx Timing"(reference=w624, error in=w623, "More:Reference Clock:Source"=w619, "More:Synchronization Pulse:Source"=w620) -> (reference out=w636:refnum<k21>, error out=w635:errorcluster)
          n167 = property class="DAQmx Timing"(reference=w628, error in=w622, "More:Reference Clock:Source"=w619, "More:Synchronization Pulse:Source"=w620) -> (reference out=w633:refnum<k21>, error out=w634:errorcluster)
          n168 = property class="DAQmx Timing"(reference=w625, error in=w621, "More:Reference Clock:Source"=w619, "More:Synchronization Pulse:Source"=w620) -> (reference out=w632:refnum<k21>, error out=w631:errorcluster)
          n169 = property class="DAQmx Timing"(reference=w626, error in=w627, "More:Reference Clock:Source"=w619, "More:Synchronization Pulse:Source"=w620) -> (reference out=w629:refnum<k21>, error out=w630:errorcluster)
        }
        frame 3 {
          n170 = property class="DAQmx Timing"(reference=w642, error in=w641, "More:Reference Clock:Source"=w637, "More:Synchronization Pulse:Source"=w638) -> (reference out=w650:refnum<k21>, error out=w649:errorcluster)
          n171 = property class="DAQmx Timing"(reference=w644, error in=w640, "More:Reference Clock:Source"=w637, "More:Synchronization Pulse:Source"=w638) -> (reference out=w647:refnum<k21>, error out=w648:errorcluster)
          n172 = property class="DAQmx Timing"(reference=w643, error in=w639, "More:Reference Clock:Source"=w637, "More:Synchronization Pulse:Source"=w638) -> (reference out=w646:refnum<k21>, error out=w645:errorcluster)
        }
        frame 2 {
          n173 = property class="DAQmx Timing"(reference=w655, error in=w654, "More:Reference Clock:Source"=w651, "More:Synchronization Pulse:Source"=w652) -> (reference out=w660:refnum<k21>, error out=w659:errorcluster)
          n174 = property class="DAQmx Timing"(reference=w656, error in=w653, "More:Reference Clock:Source"=w651, "More:Synchronization Pulse:Source"=w652) -> (reference out=w657:refnum<k21>, error out=w658:errorcluster)
        }
        frame 1 {
          n175 = property class="DAQmx Timing"(reference=w664, error in=w663, "More:Reference Clock:Source"=w661, "More:Synchronization Pulse:Source"=w662) -> (reference out=w666:refnum<k21>, error out=w665:errorcluster)
        }
      }
      n176 = case shown="4, Default" w582 {
        tunnel: w616 -> [w680 w690 w696 _]
        tunnel: w615 -> [w679 w689 w695 _]
        tunnel: [w678 w688 w694 _] -> w614
        tunnel: [w677 w687 w693 _] -> w613
        tunnel: [w676 w686 _ _] -> w612
        tunnel: [w675 w685 _ _] -> w611
        tunnel: w610 -> [w674 w684 _ _]
        tunnel: w609 -> [w673 w683 _ _]
        tunnel: w608 -> [w672 _ _ _]
        tunnel: w607 -> [w671 _ _ _]
        tunnel: [w670 _ _ _] -> w606
        tunnel: [w669 _ _ _] -> w605
        tunnel: w586 -> [w668 w682 w692 _]
        tunnel: w584 -> [w667 w681 w691 _]
        frame 4, Default {
          n177 = property class="DAQmx Timing"(reference=w680, error in=w679, "More:Reference Clock:Source"=w667, "More:Synchronization Pulse:Source"=w668) -> (reference out=w678:refnum<k21>, error out=w677:errorcluster)
          n178 = property class="DAQmx Timing"(reference=w673, error in=w674, "More:Reference Clock:Source"=w667, "More:Synchronization Pulse:Source"=w668) -> (reference out=w675:refnum<k21>, error out=w676:errorcluster)
          n179 = property class="DAQmx Timing"(reference=w672, error in=w671, "More:Reference Clock:Source"=w667, "More:Synchronization Pulse:Source"=w668) -> (reference out=w670:refnum<k21>, error out=w669:errorcluster)
        }
        frame 3 {
          n180 = property class="DAQmx Timing"(reference=w690, error in=w689, "More:Reference Clock:Source"=w681, "More:Synchronization Pulse:Source"=w682) -> (reference out=w688:refnum<k21>, error out=w687:errorcluster)
          n181 = property class="DAQmx Timing"(reference=w683, error in=w684, "More:Reference Clock:Source"=w681, "More:Synchronization Pulse:Source"=w682) -> (reference out=w685:refnum<k21>, error out=w686:errorcluster)
        }
        frame 2 {
          n182 = property class="DAQmx Timing"(reference=w696, error in=w695, "More:Reference Clock:Source"=w691, "More:Synchronization Pulse:Source"=w692) -> (reference out=w694:refnum<k21>, error out=w693:errorcluster)
        }
        frame 1 {
        }
      }
    }
    frame "USB-4431" {
      n183 = call "Get Dev Product Type.vi"("error in (no error)"=w703, "Refnum in"=w707) -> ("error out"=w699:errorcluster, "ProductType"=w704:string, "ActiveDev"=w705:tag, "Refnum out"=w706:refnum<k21>)  [unwired: 6 in]
      n184 = call "44xxRefClk.vi"("error in (no error)"=w699, "ProductType"=w704, "ActiveDev"=w705, "Refnum in"=w706) -> ("error out"=w700:errorcluster, "RefClk.Src"=w701:tag, "Refnum out"=w702:refnum<k21>)  [unwired: 5 in]
      n185 = property class="DAQmx Timing"(reference=w702, error in=w700, "More:Reference Clock:Source"=w701) -> (reference out=w697:refnum<k21>, error out=w698:errorcluster)
    }
  }
  n186 = call "Get Terminal Name with Device Prefix.vi"("error in (no error)"=w134, "Local Terminal Name"="ai/StartTrigger", "task/channels in"=w135) -> ("error out"=w132:errorcluster, "Terminal Name with Device Prefix"=w108:tag, "task out"=w133:refnum<k21>)  [unwired: 6 in]
  n187 = case shown="1" w168 {
    tunnel: w118 -> [w738 w751 w760 w765]
    tunnel: w117 -> [w737 w750 w759 w764]
    tunnel: [w736 w749 w758 w763] -> w116
    tunnel: [w735 w748 w757 w762] -> w115
    tunnel: w114 -> [w734 w747 w756 _]
    tunnel: w113 -> [w733 w746 w755 _]
    tunnel: w112 -> [w732 w745 _ _]
    tunnel: w111 -> [w731 w744 _ _]
    tunnel: w110 -> [w730 _ _ _]
    tunnel: w109 -> [w729 _ _ _]
    tunnel: w108 -> [w728 w743 w754 w761]
    tunnel: [w727 w742 w753 _] -> w40
    tunnel: [w726 w741 w752 _] -> w39
    tunnel: [w725 w740 _ _] -> w38
    tunnel: [w724 w739 _ _] -> w37
    tunnel: [w723 _ _ _] -> w36
    tunnel: [w722 _ _ _] -> w35
    frame 4, Default {
      n188 = call-poly <vilib>:"DAQmx Trigger.vi"("task/channels in"=w738, "source"=w728, "error in"=w737) -> ("task out"=w736:refnum<k21>, "error out"=w735:errorcluster)  [unwired: 11 in]
      n189 = call-poly <vilib>:"DAQmx Trigger.vi"("task/channels in"=w733, "source"=w728, "error in"=w734) -> ("task out"=w726:refnum<k21>, "error out"=w727:errorcluster)  [unwired: 11 in]
      n190 = call-poly <vilib>:"DAQmx Trigger.vi"("task/channels in"=w732, "source"=w728, "error in"=w731) -> ("task out"=w725:refnum<k21>, "error out"=w724:errorcluster)  [unwired: 11 in]
      n191 = call-poly <vilib>:"DAQmx Trigger.vi"("task/channels in"=w729, "source"=w728, "error in"=w730) -> ("task out"=w722:refnum<k21>, "error out"=w723:errorcluster)  [unwired: 11 in]
    }
    frame 3 {
      n192 = call-poly <vilib>:"DAQmx Trigger.vi"("task/channels in"=w751, "source"=w743, "error in"=w750) -> ("task out"=w749:refnum<k21>, "error out"=w748:errorcluster)  [unwired: 11 in]
      n193 = call-poly <vilib>:"DAQmx Trigger.vi"("task/channels in"=w746, "source"=w743, "error in"=w747) -> ("task out"=w741:refnum<k21>, "error out"=w742:errorcluster)  [unwired: 11 in]
      n194 = call-poly <vilib>:"DAQmx Trigger.vi"("task/channels in"=w745, "source"=w743, "error in"=w744) -> ("task out"=w740:refnum<k21>, "error out"=w739:errorcluster)  [unwired: 11 in]
    }
    frame 2 {
      n195 = call-poly <vilib>:"DAQmx Trigger.vi"("task/channels in"=w760, "source"=w754, "error in"=w759) -> ("task out"=w758:refnum<k21>, "error out"=w757:errorcluster)  [unwired: 11 in]
      n196 = call-poly <vilib>:"DAQmx Trigger.vi"("task/channels in"=w755, "source"=w754, "error in"=w756) -> ("task out"=w752:refnum<k21>, "error out"=w753:errorcluster)  [unwired: 11 in]
    }
    frame 1 {
      n197 = call-poly <vilib>:"DAQmx Trigger.vi"("task/channels in"=w765, "source"=w761, "error in"=w764) -> ("task out"=w763:refnum<k21>, "error out"=w762:errorcluster)  [unwired: 11 in]
    }
  }
  n198 = case shown="2" w6 {
    tunnel: w129 -> [w778 w787 w792 _]
    tunnel: w128 -> [w777 w786 w791 _]
    tunnel: w127 -> [w776 w785 _ _]
    tunnel: w126 -> [w775 w784 _ _]
    tunnel: w121 -> [w774 _ _ _]
    tunnel: w120 -> [w773 _ _ _]
    tunnel: w108 -> [w772 w783 w790 _]
    tunnel: [w771 _ _ _] -> w46
    tunnel: [w770 w782 _ _] -> w45
    tunnel: [w769 w781 w789 _] -> w44
    tunnel: [w768 w780 w788 _] -> w43
    tunnel: [w767 w779 _ _] -> w42
    tunnel: [w766 _ _ _] -> w41
    frame 4, Default {
      n199 = call-poly <vilib>:"DAQmx Trigger.vi"("task/channels in"=w778, "source"=w772, "error in"=w777) -> ("task out"=w769:refnum<k21>, "error out"=w768:errorcluster)  [unwired: 11 in]
      n200 = call-poly <vilib>:"DAQmx Trigger.vi"("task/channels in"=w775, "source"=w772, "error in"=w776) -> ("task out"=w770:refnum<k21>, "error out"=w767:errorcluster)  [unwired: 11 in]
      n201 = call-poly <vilib>:"DAQmx Trigger.vi"("task/channels in"=w774, "source"=w772, "error in"=w773) -> ("task out"=w771:refnum<k21>, "error out"=w766:errorcluster)  [unwired: 11 in]
    }
    frame 3 {
      n202 = call-poly <vilib>:"DAQmx Trigger.vi"("task/channels in"=w787, "source"=w783, "error in"=w786) -> ("task out"=w781:refnum<k21>, "error out"=w780:errorcluster)  [unwired: 11 in]
      n203 = call-poly <vilib>:"DAQmx Trigger.vi"("task/channels in"=w784, "source"=w783, "error in"=w785) -> ("task out"=w782:refnum<k21>, "error out"=w779:errorcluster)  [unwired: 11 in]
    }
    frame 2 {
      n204 = call-poly <vilib>:"DAQmx Trigger.vi"("task/channels in"=w792, "source"=w790, "error in"=w791) -> ("task out"=w789:refnum<k21>, "error out"=w788:errorcluster)  [unwired: 11 in]
    }
    frame 1 {
    }
  }
  n205 = case shown="\"USB-4431\"" w8 {
    tunnel: w133 -> [w838 w934]
    tunnel: w132 -> [w837 w933]
    tunnel: [w836 w933] -> w25
    tunnel: [w835 w934] -> w26
    tunnel: [w834 w932] -> w119
    tunnel: w116 -> [w833 w926]
    tunnel: w115 -> [w832 w925]
    tunnel: [w831 w930] -> w107
    tunnel: [w830 w928] -> w106
    tunnel: [w829 w931] -> w105
    tunnel: [w828 w929] -> w104
    tunnel: [w827 w927] -> w103
    tunnel: [w826 w926] -> w102
    tunnel: [w825 w924] -> w101
    tunnel: [w824 w922] -> w100
    tunnel: [w823 w925] -> w99
    tunnel: [w822 w923] -> w98
    tunnel: [w821 w921] -> w97
    tunnel: [w820 w920] -> w96
    tunnel: [w819 w919] -> w95
    tunnel: w46 -> [w818 w928]
    tunnel: w45 -> [w817 w930]
    tunnel: w44 -> [w816 w932]
    tunnel: w43 -> [w815 w931]
    tunnel: w42 -> [w814 w929]
    tunnel: w41 -> [w813 w927]
    tunnel: w40 -> [w812 w923]
    tunnel: w39 -> [w811 w924]
    tunnel: w38 -> [w810 w922]
    tunnel: w37 -> [w809 w921]
    tunnel: w36 -> [w808 w919]
    tunnel: w35 -> [w807 w920]
    tunnel: w168 -> [w794 _]
    tunnel: w6 -> [w793 _]
    frame Default {
      n206 = case shown="4, Default" w793 {
        tunnel: [w903 w913 w918 _] -> w834
        tunnel: [w902 w912 _ _] -> w831
        tunnel: [w901 _ _ _] -> w830
        tunnel: [w900 w911 w917 _] -> w829
        tunnel: [w899 w910 _ _] -> w828
        tunnel: [w898 _ _ _] -> w827
        tunnel: w818 -> [w897 _ _ _]
        tunnel: w817 -> [w896 w909 _ _]
        tunnel: w816 -> [w895 w908 w916 _]
        tunnel: w815 -> [w894 w907 w915 _]
        tunnel: w814 -> [w893 w906 _ _]
        tunnel: w813 -> [w892 _ _ _]
        tunnel: [w891 w905 w914 _] -> w801
        tunnel: [w890 w904 _ _] -> w800
        tunnel: [w889 _ _ _] -> w799
        frame 4, Default {
          n207 = property class="DAQmx Timing"(reference=w895, error in=w894) -> (reference out=w903:refnum<k21>, error out=w900:errorcluster, "SyncPulse.SyncTime"=w891:dbl)
          n208 = property class="DAQmx Timing"(reference=w896, error in=w893) -> (reference out=w902:refnum<k21>, error out=w899:errorcluster, "SyncPulse.SyncTime"=w890:dbl)
          n209 = property class="DAQmx Timing"(reference=w897, error in=w892) -> (reference out=w901:refnum<k21>, error out=w898:errorcluster, "SyncPulse.SyncTime"=w889:dbl)
        }
        frame 3 {
          n210 = property class="DAQmx Timing"(reference=w908, error in=w907) -> (reference out=w913:refnum<k21>, error out=w911:errorcluster, "SyncPulse.SyncTime"=w905:dbl)
          n211 = property class="DAQmx Timing"(reference=w909, error in=w906) -> (reference out=w912:refnum<k21>, error out=w910:errorcluster, "SyncPulse.SyncTime"=w904:dbl)
        }
        frame 2 {
          n212 = property class="DAQmx Timing"(reference=w916, error in=w915) -> (reference out=w918:refnum<k21>, error out=w917:errorcluster, "SyncPulse.SyncTime"=w914:dbl)
        }
        frame 1 {
        }
      }
      n213 = case shown="2" w794 {
        tunnel: w833 -> [w858 w873 w883 w888]
        tunnel: w832 -> [w857 w872 w882 w887]
        tunnel: [w856 w871 w881 w886] -> w826
        tunnel: [w855 w870 w880 _] -> w825
        tunnel: [w854 w869 _ _] -> w824
        tunnel: [w853 w868 w879 w885] -> w823
        tunnel: [w852 w867 w878 _] -> w822
        tunnel: [w851 w866 _ _] -> w821
        tunnel: [w850 _ _ _] -> w820
        tunnel: [w849 _ _ _] -> w819
        tunnel: w812 -> [w848 w865 w877 _]
        tunnel: w811 -> [w847 w864 w876 _]
        tunnel: w810 -> [w846 w863 _ _]
        tunnel: w809 -> [w845 w862 _ _]
        tunnel: w808 -> [w844 _ _ _]
        tunnel: w807 -> [w843 _ _ _]
        tunnel: [w842 w861 w875 w884] -> w798
        tunnel: [w841 w860 w874 _] -> w797
        tunnel: [w840 w859 _ _] -> w796
        tunnel: [w839 _ _ _] -> w795
        frame 4, Default {
          n214 = property class="DAQmx Timing"(reference=w858, error in=w857) -> (reference out=w856:refnum<k21>, error out=w853:errorcluster, "SyncPulse.SyncTime"=w842:dbl)
          n215 = property class="DAQmx Timing"(reference=w847, error in=w848) -> (reference out=w855:refnum<k21>, error out=w852:errorcluster, "SyncPulse.SyncTime"=w841:dbl)
          n216 = property class="DAQmx Timing"(reference=w846, error in=w845) -> (reference out=w854:refnum<k21>, error out=w851:errorcluster, "SyncPulse.SyncTime"=w840:dbl)
          n217 = property class="DAQmx Timing"(reference=w843, error in=w844) -> (reference out=w850:refnum<k21>, error out=w849:errorcluster, "SyncPulse.SyncTime"=w839:dbl)
        }
        frame 3 {
          n218 = property class="DAQmx Timing"(reference=w873, error in=w872) -> (reference out=w871:refnum<k21>, error out=w868:errorcluster, "SyncPulse.SyncTime"=w861:dbl)
          n219 = property class="DAQmx Timing"(reference=w864, error in=w865) -> (reference out=w870:refnum<k21>, error out=w867:errorcluster, "SyncPulse.SyncTime"=w860:dbl)
          n220 = property class="DAQmx Timing"(reference=w863, error in=w862) -> (reference out=w869:refnum<k21>, error out=w866:errorcluster, "SyncPulse.SyncTime"=w859:dbl)
        }
        frame 2 {
          n221 = property class="DAQmx Timing"(reference=w883, error in=w882) -> (reference out=w881:refnum<k21>, error out=w879:errorcluster, "SyncPulse.SyncTime"=w875:dbl)
          n222 = property class="DAQmx Timing"(reference=w876, error in=w877) -> (reference out=w880:refnum<k21>, error out=w878:errorcluster, "SyncPulse.SyncTime"=w874:dbl)
        }
        frame 1 {
          n223 = property class="DAQmx Timing"(reference=w888, error in=w887) -> (reference out=w886:refnum<k21>, error out=w885:errorcluster, "SyncPulse.SyncTime"=w884:dbl)
        }
      }
      n224 = property class="DAQmx Timing"(reference=w838, error in=w837) -> (reference out=w804:refnum<k21>, error out=w805:errorcluster, "SyncPulse.SyncTime"=w806:dbl)
      n225 = Build Array(w806, w801, w800, w799, w798, w797, w796, w795) -> (w803:dbl[])
      n226 = Array Max & Min(array=w803) -> (max value=w802:dbl)  [unwired: 3 out]
      n227 = property class="DAQmx Timing"(reference=w804, error in=w805, "SyncPulse.MinDelayToStart"=w802) -> (reference out=w835:refnum<k21>, error out=w836:errorcluster)
    }
    frame "USB-4431" {
    }
  }
  n228 = Not(x=w171) -> (.not. x?=w170:bool)
  n229 = call "4461 - Create AO waveforms.vi"("sampling info"="sampling info", "error in (no error)"="error in", "reset signal"=w170, "AO"="AO") -> ("error out"=w30:errorcluster, "AO Array"=w21:waveform(dbl)[])  [unwired: 4 in, 2 out]
  n230 = call "4461 - Create Reference Waveforms.vi"("sampling info"="sampling info", "reset signal"=w170, "Lockin"="Channels: Lockin") -> ()  [unwired: 5 in, 4 out]
  n231 = case shown="\"USB-4431\"" w8 {
    tunnel: [w943 w949] -> w90
    tunnel: [w942 w948] -> w89
    tunnel: [w941 w947] -> w88
    tunnel: [w939 w945] -> w27
    tunnel: w21 -> [w938 w944]
    frame "USB-4431" {
      n232 = Index Array(array=w938) -> (element #1=w940:waveform(dbl), element #2=w937:waveform(dbl), element #3=w936:waveform(dbl), element #4=w935:waveform(dbl))  [unwired: 4 in]
      n233 = Build Array(w940) -> (w939:waveform(dbl)[])
      n234 = Build Array(w937) -> (w943:waveform(dbl)[])
      n235 = Build Array(w936) -> (w942:waveform(dbl)[])
      n236 = Build Array(w935) -> (w941:waveform(dbl)[])
    }
    frame Default {
      n237 = Index Array(array=w944) -> (element #1=w946:waveform(dbl), element #2=w956:waveform(dbl), element #3=w955:waveform(dbl), element #4=w954:waveform(dbl), element #5=w953:waveform(dbl), element #6=w952:waveform(dbl), element #7=w951:waveform(dbl), element #8=w950:waveform(dbl))  [unwired: 8 in]
      n238 = Build Array(w946, w956) -> (w945:waveform(dbl)[])
      n239 = Build Array(w955, w954) -> (w949:waveform(dbl)[])
      n240 = Build Array(w953, w952) -> (w948:waveform(dbl)[])
      n241 = Build Array(w951, w950) -> (w947:waveform(dbl)[])
    }
  }
  n242 = flat-sequence {
    tunnel: w25 -> [w961]
    tunnel: w26 -> [w960]
    tunnel: [w961] -> w167
    tunnel: [w983] -> w166
    tunnel: w119 -> [w983]
    tunnel: [w982] -> w165
    tunnel: w107 -> [w982]
    tunnel: [w981] -> w164
    tunnel: w106 -> [w981]
    tunnel: [w980] -> w163
    tunnel: w105 -> [w980]
    tunnel: [w979] -> w162
    tunnel: w104 -> [w979]
    tunnel: [w978] -> w161
    tunnel: w103 -> [w978]
    tunnel: w102 -> [w958]
    tunnel: [w967] -> w160
    tunnel: w101 -> [w968]
    tunnel: [w971] -> w159
    tunnel: w100 -> [w970]
    tunnel: [w959] -> w158
    tunnel: w99 -> [w959]
    tunnel: w98 -> [w969]
    tunnel: [w972] -> w157
    tunnel: w97 -> [w973]
    tunnel: [w974] -> w156
    tunnel: w96 -> [w977]
    tunnel: [w975] -> w155
    tunnel: w95 -> [w976]
    tunnel: [w966] -> w154
    tunnel: w90 -> [w965]
    tunnel: w89 -> [w964]
    tunnel: w88 -> [w963]
    tunnel: w168 -> [w962]
    tunnel: w27 -> [w957]
    tunnel: [w960] -> w24
    tunnel: [w958] -> w23
    tunnel: [w957] -> w22
    tunnel: [w1032] -> w153
    tunnel: [w1031] -> w152
    tunnel: w167 -> [w1031]
    tunnel: [w1030] -> w151
    tunnel: w166 -> [w1030]
    tunnel: [w1029] -> w150
    tunnel: w165 -> [w1029]
    tunnel: [w1028] -> w149
    tunnel: w164 -> [w1028]
    tunnel: [w1027] -> w148
    tunnel: w163 -> [w1027]
    tunnel: [w1026] -> w147
    tunnel: w162 -> [w1026]
    tunnel: [w1025] -> w146
    tunnel: w161 -> [w1025]
    tunnel: [w1017] -> w145
    tunnel: [w1024] -> w144
    tunnel: w160 -> [w1024]
    tunnel: [w1023] -> w143
    tunnel: w159 -> [w1023]
    tunnel: [w1016] -> w142
    tunnel: w158 -> [w1015]
    tunnel: [w1022] -> w141
    tunnel: [w1021] -> w140
    tunnel: w157 -> [w1021]
    tunnel: [w1020] -> w139
    tunnel: w156 -> [w1020]
    tunnel: [w1019] -> w138
    tunnel: w155 -> [w1019]
    tunnel: w154 -> [w1022]
    tunnel: w24 -> [w1032]
    tunnel: w23 -> [w1018]
    tunnel: w22 -> [w1014]
    tunnel: [w1064] -> w137
    tunnel: [w1063] -> w136
    tunnel: w153 -> [w1064]
    tunnel: w152 -> [w1063]
    tunnel: w151 -> [w1062]
    tunnel: w150 -> [w1061]
    tunnel: w149 -> [w1060]
    tunnel: w148 -> [w1059]
    tunnel: w147 -> [w1058]
    tunnel: w146 -> [w1057]
    tunnel: w145 -> [w1056]
    tunnel: w144 -> [w1055]
    tunnel: w143 -> [w1054]
    tunnel: w142 -> [w1053]
    tunnel: w141 -> [w1052]
    tunnel: w140 -> [w1051]
    tunnel: w139 -> [w1050]
    tunnel: w138 -> [w1049]
    tunnel: [w1048] -> w66
    tunnel: [w1047] -> w65
    tunnel: [w1046] -> w64
    tunnel: [w1045] -> w94
    tunnel: [w1044] -> w93
    tunnel: [w1043] -> w92
    tunnel: [w1042] -> w49
    tunnel: [w1041] -> w61
    tunnel: [w1040] -> w62
    tunnel: [w1039] -> w63
    tunnel: [w1038] -> w53
    tunnel: [w1037] -> w87
    tunnel: [w1036] -> w86
    tunnel: [w1035] -> w85
    tunnel: w6 -> [w1034]
    tunnel: w168 -> [w1033]
    frame #0 {
      n243 = case shown="1" w962 {
        tunnel: w977 -> [w998 _ _ _]
        tunnel: w976 -> [w997 _ _ _]
        tunnel: [w996 _ _ _] -> w975
        tunnel: [w995 _ _ _] -> w974
        tunnel: w973 -> [w994 w1008 _ _]
        tunnel: [w993 w1007 _ _] -> w972
        tunnel: [w992 w1006 _ _] -> w971
        tunnel: w970 -> [w991 w1005 _ _]
        tunnel: w969 -> [w990 w1004 w1013 _]
        tunnel: w968 -> [w989 w1003 w1012 _]
        tunnel: [w988 w1002 w1011 _] -> w967
        tunnel: [w987 w1001 w1010 _] -> w966
        tunnel: w965 -> [w986 w1000 w1009 _]
        tunnel: w964 -> [w985 w999 _ _]
        tunnel: w963 -> [w984 _ _ _]
        frame 4, Default {
          n244 = call-poly <vilib>:"DAQmx Write.vi"("task/channels in"=w991, "data"=w985, "error in"=w994) -> ("task out"=w992:refnum<k21>, "error out"=w993:errorcluster)  [unwired: 10 in, 1 out]
          n245 = call-poly <vilib>:"DAQmx Write.vi"("task/channels in"=w998, "data"=w984, "error in"=w997) -> ("task out"=w995:refnum<k21>, "error out"=w996:errorcluster)  [unwired: 10 in, 1 out]
          n246 = call-poly <vilib>:"DAQmx Write.vi"("task/channels in"=w989, "data"=w986, "error in"=w990) -> ("task out"=w988:refnum<k21>, "error out"=w987:errorcluster)  [unwired: 10 in, 1 out]
        }
        frame 3 {
          n247 = call-poly <vilib>:"DAQmx Write.vi"("task/channels in"=w1005, "data"=w999, "error in"=w1008) -> ("task out"=w1006:refnum<k21>, "error out"=w1007:errorcluster)  [unwired: 10 in, 1 out]
          n248 = call-poly <vilib>:"DAQmx Write.vi"("task/channels in"=w1003, "data"=w1000, "error in"=w1004) -> ("task out"=w1002:refnum<k21>, "error out"=w1001:errorcluster)  [unwired: 10 in, 1 out]
        }
        frame 2 {
          n249 = call-poly <vilib>:"DAQmx Write.vi"("task/channels in"=w1012, "data"=w1009, "error in"=w1013) -> ("task out"=w1011:refnum<k21>, "error out"=w1010:errorcluster)  [unwired: 10 in, 1 out]
        }
        frame 1 {
        }
      }
    }
    frame #1 {
      n250 = call-poly <vilib>:"DAQmx Write.vi"("task/channels in"=w1018, "data"=w1014, "error in"=w1015) -> ("task out"=w1017:refnum<k21>, "error out"=w1016:errorcluster)  [unwired: 10 in, 1 out]
    }
    frame #2 {
      n251 = case shown="3" w1034 {
        tunnel: w1062 -> [w1116 w1124 w1128 _]
        tunnel: w1061 -> [w1115 w1123 _ _]
        tunnel: w1060 -> [w1114 _ _ _]
        tunnel: w1059 -> [w1113 w1122 w1127 _]
        tunnel: w1058 -> [w1112 w1121 _ _]
        tunnel: w1057 -> [w1111 _ _ _]
        tunnel: [w1110 w1120 w1126 _] -> w1048
        tunnel: [w1109 w1119 _ _] -> w1047
        tunnel: [w1108 _ _ _] -> w1046
        tunnel: [w1107 w1118 w1125 _] -> w1041
        tunnel: [w1106 w1117 _ _] -> w1040
        tunnel: [w1105 _ _ _] -> w1039
        frame 4, Default {
          n252 = call <vilib>:"DAQmx Start Task.vi"("task/channels in"=w1116, "error in"=w1113) -> ("task out"=w1110:refnum<k21>, "error out"=w1107:errorcluster)  [unwired: 12 in]
          n253 = call <vilib>:"DAQmx Start Task.vi"("task/channels in"=w1115, "error in"=w1112) -> ("task out"=w1109:refnum<k21>, "error out"=w1106:errorcluster)  [unwired: 12 in]
          n254 = call <vilib>:"DAQmx Start Task.vi"("task/channels in"=w1114, "error in"=w1111) -> ("task out"=w1108:refnum<k21>, "error out"=w1105:errorcluster)  [unwired: 12 in]
        }
        frame 3 {
          n255 = call <vilib>:"DAQmx Start Task.vi"("task/channels in"=w1124, "error in"=w1122) -> ("task out"=w1120:refnum<k21>, "error out"=w1118:errorcluster)  [unwired: 12 in]
          n256 = call <vilib>:"DAQmx Start Task.vi"("task/channels in"=w1123, "error in"=w1121) -> ("task out"=w1119:refnum<k21>, "error out"=w1117:errorcluster)  [unwired: 12 in]
        }
        frame 2 {
          n257 = call <vilib>:"DAQmx Start Task.vi"("task/channels in"=w1128, "error in"=w1127) -> ("task out"=w1126:refnum<k21>, "error out"=w1125:errorcluster)  [unwired: 12 in]
        }
        frame 1 {
        }
      }
      n258 = case shown="1" w1033 {
        tunnel: w1056 -> [w1080 w1092 w1100 w1104]
        tunnel: w1055 -> [w1079 w1091 w1099 _]
        tunnel: w1054 -> [w1078 w1090 _ _]
        tunnel: w1053 -> [w1077 w1089 w1098 w1103]
        tunnel: w1052 -> [w1076 w1088 w1097 _]
        tunnel: w1051 -> [w1075 w1087 _ _]
        tunnel: w1050 -> [w1074 _ _ _]
        tunnel: w1049 -> [w1073 _ _ _]
        tunnel: [w1072 w1086 w1096 w1102] -> w1045
        tunnel: [w1071 w1085 w1095 _] -> w1044
        tunnel: [w1070 w1084 _ _] -> w1043
        tunnel: [w1069 _ _ _] -> w1042
        tunnel: [w1068 w1083 w1094 w1101] -> w1038
        tunnel: [w1067 w1082 w1093 _] -> w1037
        tunnel: [w1066 w1081 _ _] -> w1036
        tunnel: [w1065 _ _ _] -> w1035
        frame 4, Default {
          n259 = call <vilib>:"DAQmx Start Task.vi"("task/channels in"=w1080, "error in"=w1077) -> ("task out"=w1072:refnum<k21>, "error out"=w1068:errorcluster)  [unwired: 12 in]
          n260 = call <vilib>:"DAQmx Start Task.vi"("task/channels in"=w1079, "error in"=w1076) -> ("task out"=w1071:refnum<k21>, "error out"=w1067:errorcluster)  [unwired: 12 in]
          n261 = call <vilib>:"DAQmx Start Task.vi"("task/channels in"=w1078, "error in"=w1075) -> ("task out"=w1070:refnum<k21>, "error out"=w1066:errorcluster)  [unwired: 12 in]
          n262 = call <vilib>:"DAQmx Start Task.vi"("task/channels in"=w1074, "error in"=w1073) -> ("task out"=w1069:refnum<k21>, "error out"=w1065:errorcluster)  [unwired: 12 in]
        }
        frame 3 {
          n263 = call <vilib>:"DAQmx Start Task.vi"("task/channels in"=w1092, "error in"=w1089) -> ("task out"=w1086:refnum<k21>, "error out"=w1083:errorcluster)  [unwired: 12 in]
          n264 = call <vilib>:"DAQmx Start Task.vi"("task/channels in"=w1091, "error in"=w1088) -> ("task out"=w1085:refnum<k21>, "error out"=w1082:errorcluster)  [unwired: 12 in]
          n265 = call <vilib>:"DAQmx Start Task.vi"("task/channels in"=w1090, "error in"=w1087) -> ("task out"=w1084:refnum<k21>, "error out"=w1081:errorcluster)  [unwired: 12 in]
        }
        frame 2 {
          n266 = call <vilib>:"DAQmx Start Task.vi"("task/channels in"=w1100, "error in"=w1098) -> ("task out"=w1096:refnum<k21>, "error out"=w1094:errorcluster)  [unwired: 12 in]
          n267 = call <vilib>:"DAQmx Start Task.vi"("task/channels in"=w1099, "error in"=w1097) -> ("task out"=w1095:refnum<k21>, "error out"=w1093:errorcluster)  [unwired: 12 in]
        }
        frame 1 {
          n268 = call <vilib>:"DAQmx Start Task.vi"("task/channels in"=w1104, "error in"=w1103) -> ("task out"=w1102:refnum<k21>, "error out"=w1101:errorcluster)  [unwired: 12 in]
        }
      }
    }
  }
  n269 = call <vilib>:"DAQmx Start Task.vi"("task/channels in"=w137, "error in"=w136) -> ("task out"=w67:refnum<k21>, "error out"=w47:errorcluster)  [unwired: 12 in]
  n270 = while {
    tunnel: w67 -> [w1147]
    tunnel: w47 -> [w1146]
    tunnel: [w1130] -> w54
    tunnel: [w1145] -> w68
    tunnel: w66 -> [w1144]
    tunnel: w65 -> [w1142]
    tunnel: w64 -> [w1143]
    tunnel: w63 -> [w1141]
    tunnel: w62 -> [w1140]
    tunnel: w61 -> [w1139]
    tunnel: w4 -> [w1138]
    tunnel: [w1137] -> w60
    tunnel: [w1131] -> w59
    tunnel: [w1136] -> w58
    tunnel: [w1133] -> w57
    tunnel: [w1135] -> w56
    tunnel: [w1134] -> w55
    tunnel: w6 -> [w1129]
    stop <- w1132 stop-if-true
    n271 = case shown="1" w1129 {
      tunnel: w1147 -> [w1174 w1195 w1210 w1219]
      tunnel: w1146 -> [w1173 w1194 w1209 w1218]
      tunnel: [w1172 w1193 w1208 w1217] -> w1145
      tunnel: w1144 -> [w1171 w1192 w1207 _]
      tunnel: w1143 -> [w1170 _ _ _]
      tunnel: w1142 -> [w1169 w1191 _ _]
      tunnel: w1141 -> [w1168 _ _ _]
      tunnel: w1140 -> [w1167 w1190 _ _]
      tunnel: w1139 -> [w1166 w1189 w1206 _]
      tunnel: w1138 -> [w1165 w1188 w1205 w1216]
      tunnel: [w1160 w1184 w1202 _] -> w1137
      tunnel: [w1159 w1183 _ _] -> w1136
      tunnel: [w1158 _ _ _] -> w1135
      tunnel: [w1157 _ _ _] -> w1134
      tunnel: [w1156 w1182 _ _] -> w1133
      tunnel: [w1155 w1181 w1201 w1214] -> w1132
      tunnel: [w1154 w1180 w1200 _] -> w1131
      tunnel: [w1153 w1179 w1199 w1213] -> w1130
      frame 4, Default {
        n272 = property class="DAQmx Read"(reference=w1174, error in=w1173) -> (reference out=w1172:refnum<k21>, error out=w1153:errorcluster, "AvailSampPerChan"=w1151:u32)
        n273 = property class="DAQmx Read"(reference=w1171, error in=w1166) -> (reference out=w1160:refnum<k21>, error out=w1154:errorcluster, "AvailSampPerChan"=w1150:u32)
        n274 = property class="DAQmx Read"(reference=w1169, error in=w1167) -> (reference out=w1159:refnum<k21>, error out=w1156:errorcluster, "AvailSampPerChan"=w1149:u32)
        n275 = property class="DAQmx Read"(reference=w1170, error in=w1168) -> (reference out=w1158:refnum<k21>, error out=w1157:errorcluster, "AvailSampPerChan"=w1148:u32)
        n276 = Greater Or Equal?(x=w1151, y=w1165) -> (x >= y?=w1164:bool)
        n277 = Greater Or Equal?(x=w1150, y=w1165) -> (x >= y?=w1163:bool)
        n278 = Greater Or Equal?(x=w1149, y=w1165) -> (x >= y?=w1162:bool)
        n279 = Greater Or Equal?(x=w1148, y=w1165) -> (x >= y?=w1161:bool)
        n280 = Compound Arithmetic op=AND(w1164, w1163, w1162, w1161) -> (w1152:bool)
        n281 = Compound Arithmetic op=OR(w1153, w1154, w1156, w1157, w1152) -> (w1155:bool)
      }
      frame 3 {
        n282 = property class="DAQmx Read"(reference=w1195, error in=w1194) -> (reference out=w1193:refnum<k21>, error out=w1179:errorcluster, "AvailSampPerChan"=w1177:u32)
        n283 = property class="DAQmx Read"(reference=w1192, error in=w1189) -> (reference out=w1184:refnum<k21>, error out=w1180:errorcluster, "AvailSampPerChan"=w1176:u32)
        n284 = property class="DAQmx Read"(reference=w1191, error in=w1190) -> (reference out=w1183:refnum<k21>, error out=w1182:errorcluster, "AvailSampPerChan"=w1175:u32)
        n285 = Greater Or Equal?(x=w1177, y=w1188) -> (x >= y?=w1187:bool)
        n286 = Greater Or Equal?(x=w1176, y=w1188) -> (x >= y?=w1186:bool)
        n287 = Greater Or Equal?(x=w1175, y=w1188) -> (x >= y?=w1185:bool)
        n288 = Compound Arithmetic op=AND(w1187, w1186, w1185) -> (w1178:bool)
        n289 = Compound Arithmetic op=OR(w1179, w1180, w1182, w1178) -> (w1181:bool)
      }
      frame 2 {
        n290 = property class="DAQmx Read"(reference=w1210, error in=w1209) -> (reference out=w1208:refnum<k21>, error out=w1199:errorcluster, "AvailSampPerChan"=w1197:u32)
        n291 = property class="DAQmx Read"(reference=w1207, error in=w1206) -> (reference out=w1202:refnum<k21>, error out=w1200:errorcluster, "AvailSampPerChan"=w1196:u32)
        n292 = Greater Or Equal?(x=w1197, y=w1205) -> (x >= y?=w1204:bool)
        n293 = Greater Or Equal?(x=w1196, y=w1205) -> (x >= y?=w1203:bool)
        n294 = Compound Arithmetic op=AND(w1204, w1203) -> (w1198:bool)
        n295 = Compound Arithmetic op=OR(w1199, w1200, w1198) -> (w1201:bool)
      }
      frame 1 {
        n296 = property class="DAQmx Read"(reference=w1219, error in=w1218) -> (reference out=w1217:refnum<k21>, error out=w1213:errorcluster, "AvailSampPerChan"=w1211:u32)
        n297 = Greater Or Equal?(x=w1211, y=w1216) -> (x >= y?=w1215:bool)
        n298 = Compound Arithmetic op=AND(w1215) -> (w1212:bool)
        n299 = Compound Arithmetic op=OR(w1213, w1212) -> (w1214:bool)
      }
    }
  }
  n300 = case shown="3" w6 {
    tunnel: [w1238 w1253 w1264 w1271] -> w189
    tunnel: w68 -> [w1237 w1252 w1263 w1270]
    tunnel: w60 -> [w1236 w1251 w1262 _]
    tunnel: w59 -> [w1235 w1250 w1261 _]
    tunnel: w58 -> [w1234 w1249 _ _]
    tunnel: w57 -> [w1233 w1248 _ _]
    tunnel: w56 -> [w1232 _ _ _]
    tunnel: w55 -> [w1231 _ _ _]
    tunnel: w54 -> [w1230 w1247 w1260 w1269]
    tunnel: w4 -> [w1222 w1241 w1256 w1267]
    tunnel: [w1220 w1239 w1254 w1265] -> w31
    frame 4, Default {
      n301 = call-poly <vilib>:"DAQmx Read.vi"("task/channels in"=w1237, "number of samples per channel"=w1222, "error in"=w1230) -> ("task out"=w1229:refnum<k21>, "error out"=w1221:errorcluster)  [unwired: 10 in, 1 out]
      n302 = call-poly <vilib>:"DAQmx Read.vi"("task/channels in"=w1236, "number of samples per channel"=w1222, "error in"=w1235) -> ("task out"=w1228:refnum<k21>, "error out"=w1227:errorcluster)  [unwired: 10 in, 1 out]
      n303 = call-poly <vilib>:"DAQmx Read.vi"("task/channels in"=w1234, "number of samples per channel"=w1222, "error in"=w1233) -> ("task out"=w1223:refnum<k21>, "error out"=w1226:errorcluster)  [unwired: 10 in, 1 out]
      n304 = call-poly <vilib>:"DAQmx Read.vi"("task/channels in"=w1232, "number of samples per channel"=w1222, "error in"=w1231) -> ("task out"=w1224:refnum<k21>, "error out"=w1225:errorcluster)  [unwired: 10 in, 1 out]
      n305 = Build Array(w1229, w1228, w1223, w1224) -> (w1238:refnum<k21>[])
      n306 = Merge Errors(w1221, w1227, w1226, w1225) -> (w1220:errorcluster)
    }
    frame 3 {
      n307 = call-poly <vilib>:"DAQmx Read.vi"("task/channels in"=w1252, "number of samples per channel"=w1241, "error in"=w1247) -> ("task out"=w1246:refnum<k21>, "error out"=w1240:errorcluster)  [unwired: 10 in, 1 out]
      n308 = call-poly <vilib>:"DAQmx Read.vi"("task/channels in"=w1251, "number of samples per channel"=w1241, "error in"=w1250) -> ("task out"=w1245:refnum<k21>, "error out"=w1244:errorcluster)  [unwired: 10 in, 1 out]
      n309 = call-poly <vilib>:"DAQmx Read.vi"("task/channels in"=w1249, "number of samples per channel"=w1241, "error in"=w1248) -> ("task out"=w1242:refnum<k21>, "error out"=w1243:errorcluster)  [unwired: 10 in, 1 out]
      n310 = Build Array(w1246, w1245, w1242) -> (w1253:refnum<k21>[])
      n311 = Merge Errors(w1240, w1244, w1243) -> (w1239:errorcluster)
    }
    frame 2 {
      n312 = call-poly <vilib>:"DAQmx Read.vi"("task/channels in"=w1263, "number of samples per channel"=w1256, "error in"=w1260) -> ("task out"=w1259:refnum<k21>, "error out"=w1255:errorcluster)  [unwired: 10 in, 1 out]
      n313 = call-poly <vilib>:"DAQmx Read.vi"("task/channels in"=w1262, "number of samples per channel"=w1256, "error in"=w1261) -> ("task out"=w1258:refnum<k21>, "error out"=w1257:errorcluster)  [unwired: 10 in, 1 out]
      n314 = Build Array(w1259, w1258) -> (w1264:refnum<k21>[])
      n315 = Merge Errors(w1255, w1257) -> (w1254:errorcluster)
    }
    frame 1 {
      n316 = call-poly <vilib>:"DAQmx Read.vi"("task/channels in"=w1270, "number of samples per channel"=w1267, "error in"=w1269) -> ("task out"=w1268:refnum<k21>, "error out"=w1266:errorcluster)  [unwired: 10 in, 1 out]
      n317 = Build Array(w1268) -> (w1271:refnum<k21>[])
      n318 = Merge Errors(w1266) -> (w1265:errorcluster)
    }
  }
  "AI task" <- w189
  n319 = case shown="4, Default" w168 {
    tunnel: w94 -> [w1281 w1289 w1295 w1299]
    tunnel: w93 -> [w1280 w1288 w1294 _]
    tunnel: w92 -> [w1279 w1287 _ _]
    tunnel: [w1278 w1286 w1293 w1298] -> w188
    tunnel: w87 -> [w1277 w1285 w1292 _]
    tunnel: w86 -> [w1276 w1284 _ _]
    tunnel: w85 -> [w1275 _ _ _]
    tunnel: w53 -> [w1274 w1283 w1291 w1297]
    tunnel: [w1273 w1282 w1290 w1296] -> w50
    tunnel: w49 -> [w1272 _ _ _]
    frame 4, Default {
      n320 = Build Array(w1281, w1280, w1279, w1272) -> (w1278:refnum<k21>[])
      n321 = Merge Errors(w1274, w1277, w1276, w1275) -> (w1273:errorcluster)
    }
    frame 3 {
      n322 = Build Array(w1289, w1288, w1287) -> (w1286:refnum<k21>[])
      n323 = Merge Errors(w1283, w1285, w1284) -> (w1282:errorcluster)
    }
    frame 2 {
      n324 = Build Array(w1295, w1294) -> (w1293:refnum<k21>[])
      n325 = Merge Errors(w1291, w1292) -> (w1290:errorcluster)
    }
    frame 1 {
      n326 = Build Array(w1299) -> (w1298:refnum<k21>[])
      n327 = Merge Errors(w1297) -> (w1296:errorcluster)
    }
  }
  "AO Task" <- w188
  n328 = Merge Errors(w31, w50, w30) -> (→"error out":errorcluster)
